vi "WHD_VEten_0.1.2_WS_BIDIREC_update_it-0065.vi"() -> ()   [LabVIEW 2015]
uses:
  <vilib>/LabVIEW Targets/FPGA/cRIO/shared/nicrio_ModuleControls/nicrio_cRIO-9234_DataRatesRing2.ctl
  <vilib>/RTwatchdog.llb/Watchdog expiration actions.ctl
  <vilib>/userdefined/High Color/nirio_resource_hc.ctl
  <vilib>/FPGAPlugInAG/cRIO-9031/niLvFpga_Open_cRIO-9031.vi
  <vilib>/Utility/file.llb/Write Delimited Spreadsheet (string).vi
  <vilib>/FPGAPlugInAG/cRIO-9031/niLvFpga_Run_cRIO-9031.vi
  <vilib>/Utility/error.llb/Error Cluster From Error Code.vi
  <vilib>/rvi/errors/niLvFpgaAdjustHostInterfaceError.vi
  <vilib>/rvi/interface/common/niFpgaWaitOnOcc.vi
  <vilib>/FPGAPlugInAG/cRIO-9031/niLvFpga_Reset_cRIO-9031.vi
  <vilib>/FPGAPlugInAG/cRIO-9031/niLvFpga_Close_cRIO-9031.vi
  <vilib>/rvi/interface/nirviOpenFPGA/nirviOpenFPGA.xnode
  FPGA Bitfiles/W&RDEuskotrenIBA_FPGATarget2_FPGA8a2wsBIdirec_MwruJOs6jio.lvbitx
  <vilib>/rvi/interface/nirviMethod/nirviMethod.xnode
  <vilib>/rvi/interface/nirviReadWriteControl/nirviReadWriteControl.xnode
  <vilib>/rvi/interface/nirviCloseFPGA/nirviCloseFPGA.xnode
  <vilib>/NI_Real-Time Target Support.lvlib
  AURA_Wheel/Json2Labv.lvlib
  AURA_Wheel/AuraWheelAPI/AuraWheel.lvlib
  NiFpgaLv.dll
  <vilib>/rvi/errors/niLvFpgaMergeErrorWithErrorCode.vi
  <vilib>/nisyscfg/nisyscfg.lvlib
  <vilib>/FPGAPlugInAG/cRIO-9031/niLvFpga_ConfigureFifo_cRIO-9031.vi
  <vilib>/FPGAPlugInAG/cRIO-9031/niLvFpga_StartFifo_cRIO-9031.vi
  <vilib>/FPGAPlugInAG/cRIO-9031/niLvFpga_ReadFifo_cRIO-9031.vi
  <vilib>/FPGAPlugInAG/cRIO-9031/niLvFpga_StopFifo_cRIO-9031.vi
panel:
  out "hora max subida datos":string
  out "hora subida datos":string
  in  "LIMITE MIN":dbl
  in  "LIMITE MAX":dbl
  in  "Parametros AuraWheel Health":string[](array[string])=["nem1234", "test_rest", "http://api.aurawheel.dev/services/devices/status"]
  out "Problema WS":bool
  out "Direccion 0?":bool
  out "Boton Adquirir?":bool
  out "RuedaDetectada2?":bool=TRUE
  out "RuedaDetectada1?":bool=TRUE
  in  "Timeout ruedas":dbl
  in  "Borrar archivos\nadquisicion con error":bool
  out "Watchdog config":T1={"reset"=FALSE, "occurrence"=FALSE, "trigger protocol"=enum."active high", "trigger line"=enum."none", "disable watchdog on VI exit"=TRUE}
  in  "Disable watchdog?":bool
  in  "Reset watchdog?":bool
  in  "Leer config RFID NEM":bool
  in  "bytes to read":i32
  in  "DeviceAddress":u8
  in  "timeout ms (60000)":i32
  in  "Max archivos":u32=2
  in  "Bytes libre despues de borrar":u32=2
  in  "Bytes min libre":u32=2
  in  "Nº de acelerómetros":i32
  in  "Nº inductivos":i32
  in  "Offset_rueda WS 1":fxp<+/-,24,-4>=0.004999998956918716 format="%.27g"
  out "TAGs_AURAwheel":string[][](array[string])
  out "Plataformas?":bool
  out "Nº Ejes":i32[](array[numeric])
  out "Nº UTs":i32
  out "it-read-LR6":i32[](array[numeric])
  out "it-LR6":i32
  out "RFID_LR6_Error":errorcluster
  out "Series_flota":string[](array[string])
  out "Tabla_flota":string[][](array[string])
  out "Puntos medios de las ventanas":dbl[][](array[numeric])
  out "configuration file path":path=path "c:/Parametros.cfg"
  in  "IP synchr":string
  out "data":cluster{"status":string}
  out "confRFID":path=path "c:/RFID/TAGS.csv"
  out "TAGS leidos":path=path "c:/RFID/TAGS.csv"
  in  "Use Aura?":bool
  in  "Parametros AuraWheel":string[](array[string])
  in  "Parámetros acelerómetros":dbl[](array[numeric])
  in  "Tiempo de adquisicion":dbl=10.0
  in  "Adquirir":bool
  out "Fin":bool
  out "Contador":i32=1
  out "Path TEST":path=path "c:/TEST"
  out "Fallo det presencia":bool
  out "Path_Borrar":path=path "c:/Trenes"
  out "Longitud de la unidad":dbl
  out "Bucle Espera":i32
  out "Aviso no detección":string
  out "Time to Acquire Block (ms)":i32
  out "Distancia de acelerómetros":dbl[](array[numeric])
  out "Block Size":u32
  out "Distancias generales":dbl[](array[numeric])
  in  "Reset del controlador":bool
  in  "Configuración":bool
  in  "Parar la aplicación":bool
  out "RFID":bool=TRUE
  out "date/time string":string
  out "Timeout ruedas":bool
  out "Tiempo":dbl
  out "Inicio pasada":timestamp
  out "Ultimo TEST":timestamp
  out "Fuente":bool=TRUE
  out "Estado":string
  out "RFID_ID":refnum<k5>
  out "DC OK":string
  out "Aviso temperatura":string
  in  "Tab Control":T2(tab)=enum."Parámetros"
  out "V (m/s)":dbl
  out "Temperatura (ºC)":dbl
  out "Max RMS Ruedas":dbl[][](array[numeric])
  out "result":bool
  out "TAGs":string[](array[string])
  out "Parar":bool
  out "TAGs LR6":string[](array[string])
  out "TAGs HEX":string[](array[string])
  out "Waveform Graph":sgl[][](graph)
  out "Nombre de archivo":path[](array[path])
  out "Tiempo de paso (s)":dbl
  out "Tiempo extra de adquisición (s)":dbl
  out "Número de ejes detectados":i32
  out "Buffer Underflow":bool
  out "Buffer Overflow":bool
  out "Disco Duro Disponible (bytes)":i64
  out "created path":path
  out "Nº Ruedas 1":i32
  out "NºRuedas 2":i32
  out "deleted portion":sgl[](array[numeric])
  out "deleted portion 2":sgl[](array[numeric])
  out "Ejes_convoy":i32
  out "T fuera rango":bool
  in  "Frecuencia de muestreo (Hz)":dbl=25600.0
  in  "Escaneos de la FIFO por canal":u32=5000
  in  "Tiempo extra al detector de paso (s)":dbl=1.0
  in  "dt RMS":dbl=256.0
  in  "Frecuencia de muestreo y módulo CRIO":T3=2 items=["51.200 kS/s (NI 9234)"=1, "25.600 kS/s (NI 9234)"=2, "17.067 kS/s (NI 9234)"=3, "12.800 kS/s (NI 9234)"=4, "10.240 kS/s (NI 9234)"=5, "8.533 kS/s (NI 9234)"=6, "7.314 kS/s (NI 9234)"=7, "6.400 kS/s (NI 9234)"=8, "5.689 kS/s (NI 9234)"=9, "5.120 kS/s (NI 9234)"=10, "4.654 kS/s (NI 9234)"=11, "4.267 kS/s (NI 9234)"=12, "3.938 kS/s (NI 9234)"=13, "3.657 kS/s (NI 9234)"=14, "3.413 kS/s (NI 9234)"=15, "3.200 kS/s (NI 9234)"=16, "3.012 kS/s (NI 9234)"=17, "2.845 kS/s (NI 9234)"=18, "2.695 kS/s (NI 9234)"=19, "2.560 kS/s (NI 9234)"=20, "2.438 kS/s (NI 9234)"=21, "2.328 kS/s (NI 9234)"=22, "2.226 kS/s (NI 9234)"=23, "2.133 kS/s (NI 9234)"=24, "2.048 kS/s (NI 9234)"=25, "1.969 kS/s (NI 9234)"=26, "1.896 kS/s (NI 9234)"=27, "1.829 kS/s (NI 9234)"=28, "1.765 kS/s (NI 9234)"=29, "1.707 kS/s (NI 9234)"=30, "1.652 kS/s (NI 9234)"=31]
  in  "Puerto RFID":u16=2189
  in  "IP RFID":string="192.168.106.99"
  in  "Offset_rueda WS 2":fxp<+/-,24,-4>=0.004999998956918716 format="%.27g"
  in  "Count(mSec)":u32=2
  in  "LR6 IP address":string="192.168.106.94"
  in  "Port LR6":u16=2001
  in  "RFID NEM on?":bool
  in  "RFID LR6 on?":bool
  in  "Canal cero WS1?":bool
  in  "Canal cero WS2":bool
  out "Parámetros":bool=TRUE
  out "Distacias y medidas de dispositivos":bool=TRUE
  out "RFID_Error":errorcluster
  out "error FPGA":errorcluster
  out "error manipulacion archivos":errorcluster
  out "Unidades y ejes":bool=TRUE
  out "RFID":bool=TRUE
  out "error AURA":errorcluster
  out "Response headers":string
  in  "Array":path[](array[path])=[path "c:/Trenes_prueba/0207_2013-09-24_19-09-42_0.bin", path "c:/Trenes_prueba/0096_2013-10-30_18-13-14_0.bin", path "c:/Trenes_prueba/0001_2013-06-05_13-06-23_0.bin"]
  out "Numeric 3":i32
  in  "Digital?":bool=TRUE
  # "Funciona?"
  # "Última detección de unidad"
  # "Error!!"
  # "Estado de la memoria"
  # "Parámetros de muestreo"
  # "Parámetros de adquisición"
  # "Parámetros de procesado"
  # "Cambio Fecha y Hora"
  # "Cargar datos de configuración"
  # "Errores!!"
  # "WRD_MEX\nWRD_ZAR"
  # "0 tagMexInit\n1 tagMexFin\n\n0 tag1\n1 tag2"
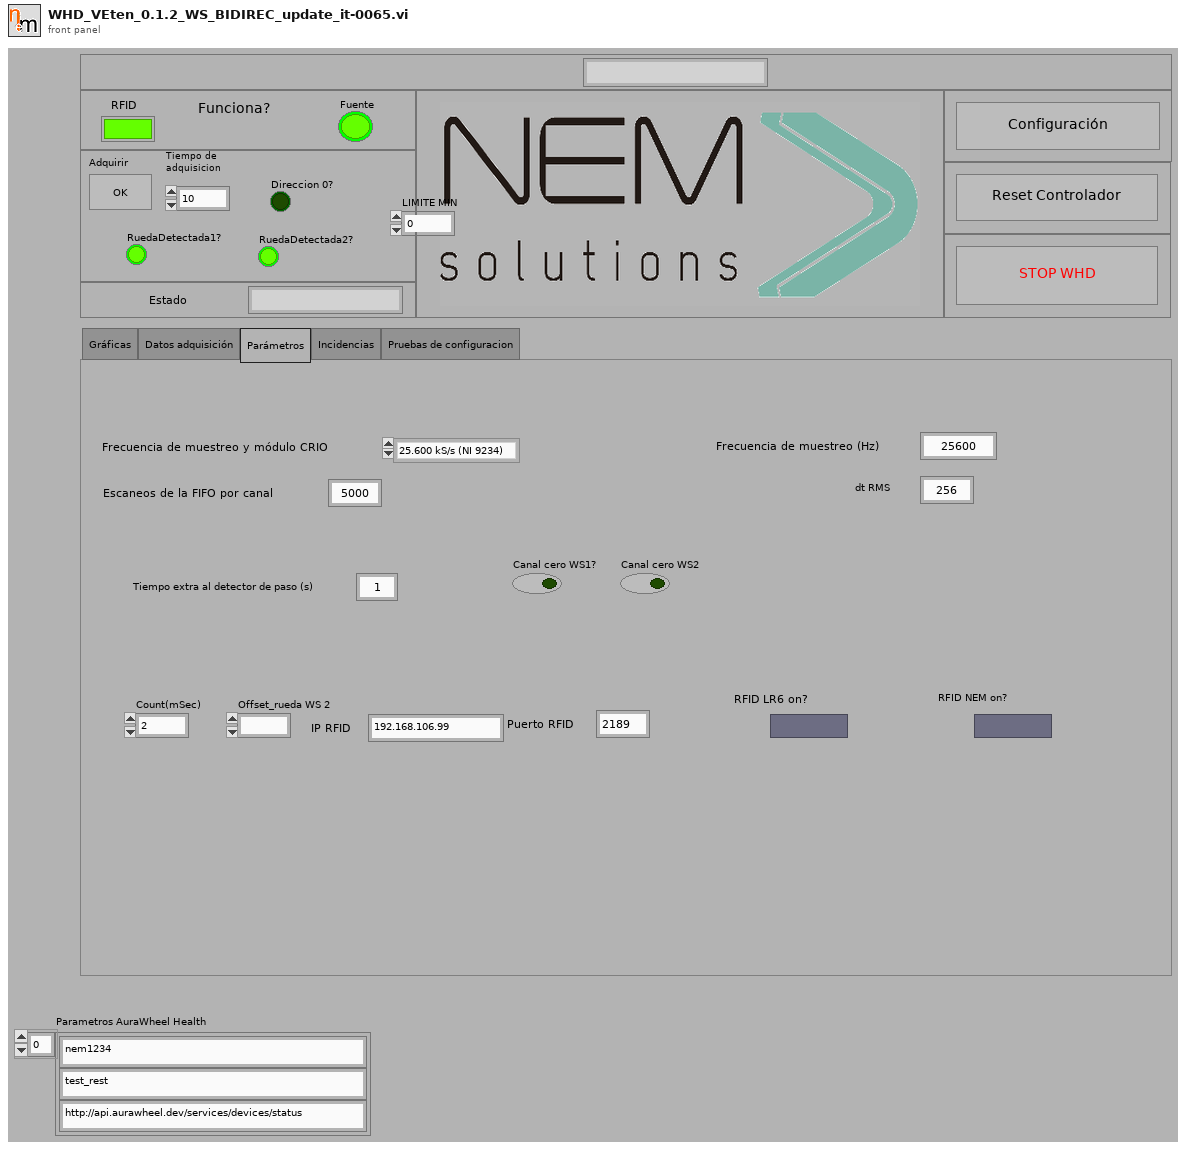
[diagram p1: front panel]
types:
  T1 = typedef "Watchdog expiration actions.ctl" = cluster{"reset":bool, "occurrence":bool, "trigger protocol":enum16{"active high", "active low", "open collector"}, "trigger line":enum16{"none", "line 0", "line 1", "line 2", "line 3", "line 4", "line 5", "line 6", "line 7", "SMB line 0"}, "disable watchdog on VI exit":bool}
  T2 = enum32{"Gráficas", "Datos adquisición", "Parámetros", "Incidencias", "Pruebas de configuracion"}
  T3 = typedef "nicrio_cRIO-9234_DataRatesRing2.ctl" = u8
  T4 = typedef "nirio_resource_hc.ctl" = tag
  T5 = enum16{"Standard", "Buffered", "CRLF", "Immediate"}
  T6 = enum16{"open", "replace", "create", "open or create", "replace or create", "replace or create with confirmation"}
  T7 = enum16{"big-endian, network order", "native, host order", "little-endian"}
  T8 = cluster{"error IO":errorcluster, bool[], u32[], string[], dbl[]}
  T9 = cluster{"g_ts":dbl, "p_sp":dbl, "p_tp":dbl, "p_tg":cluster{"tg_n":dbl, "tg_t":string}[], "p_ax":cluster{"ax_n":dbl, "ax_sp":dbl, "ax_wh":cluster{"wh_p":dbl, "wh_a1":dbl, "wh_a2":dbl, "wh_a3":dbl, "wh_a4":dbl}[]}[]}
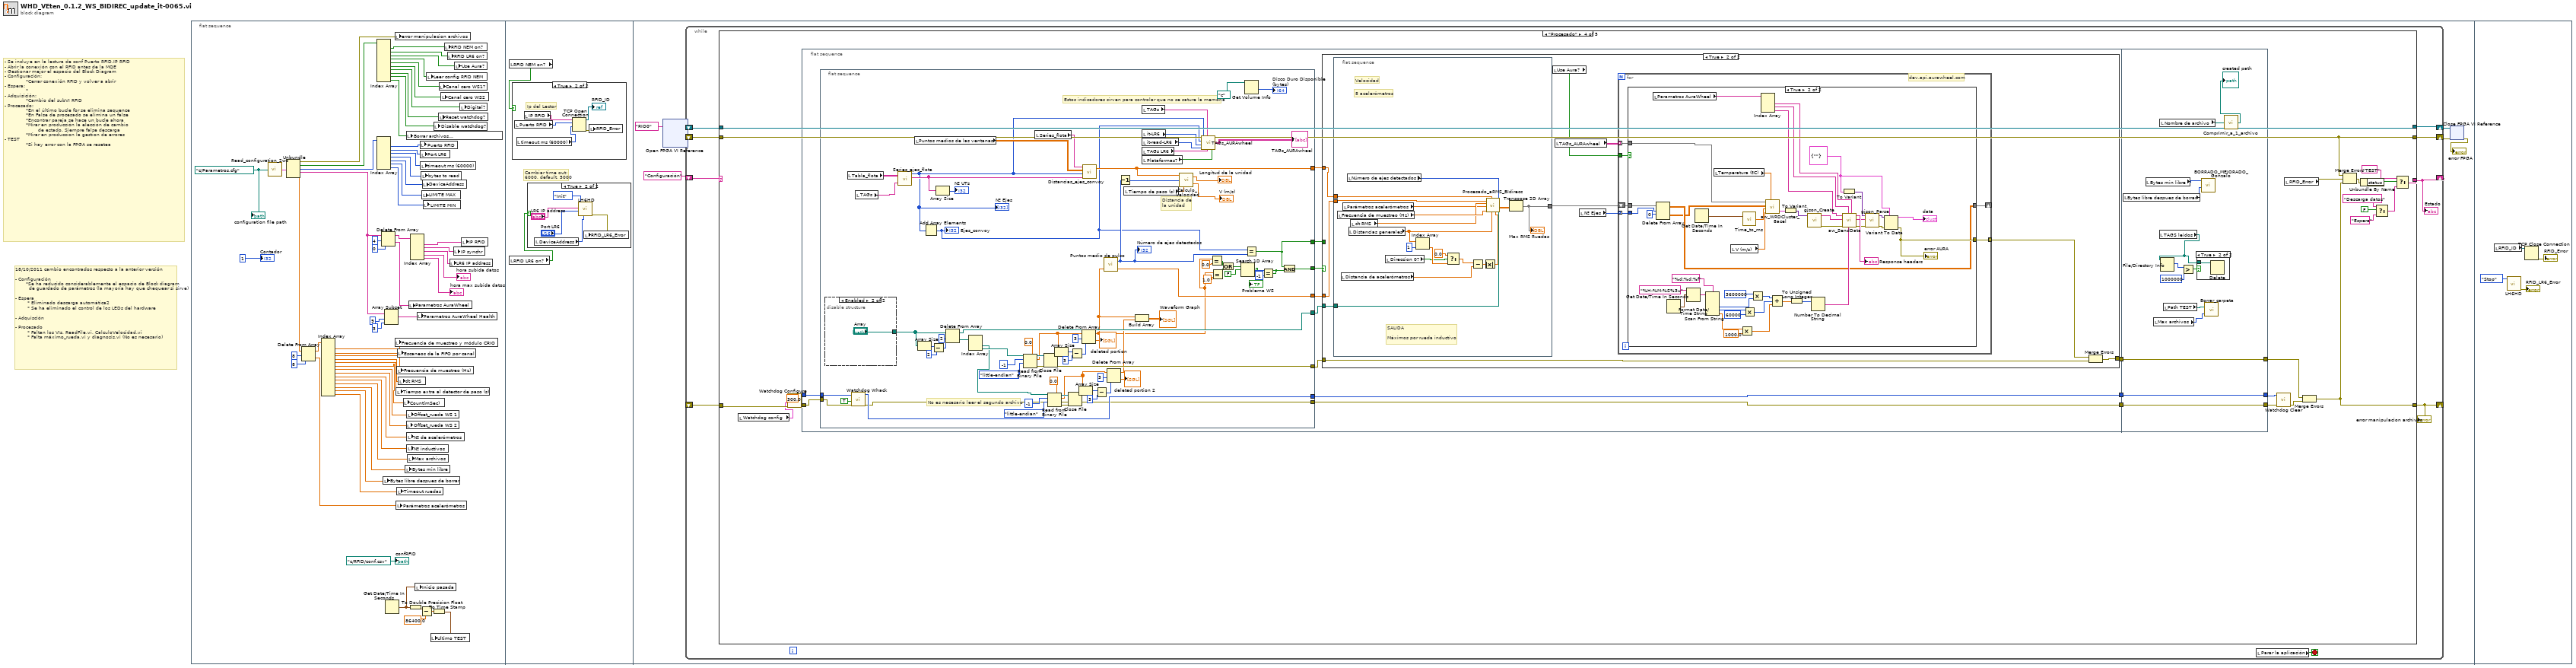
[diagram p0: block diagram]
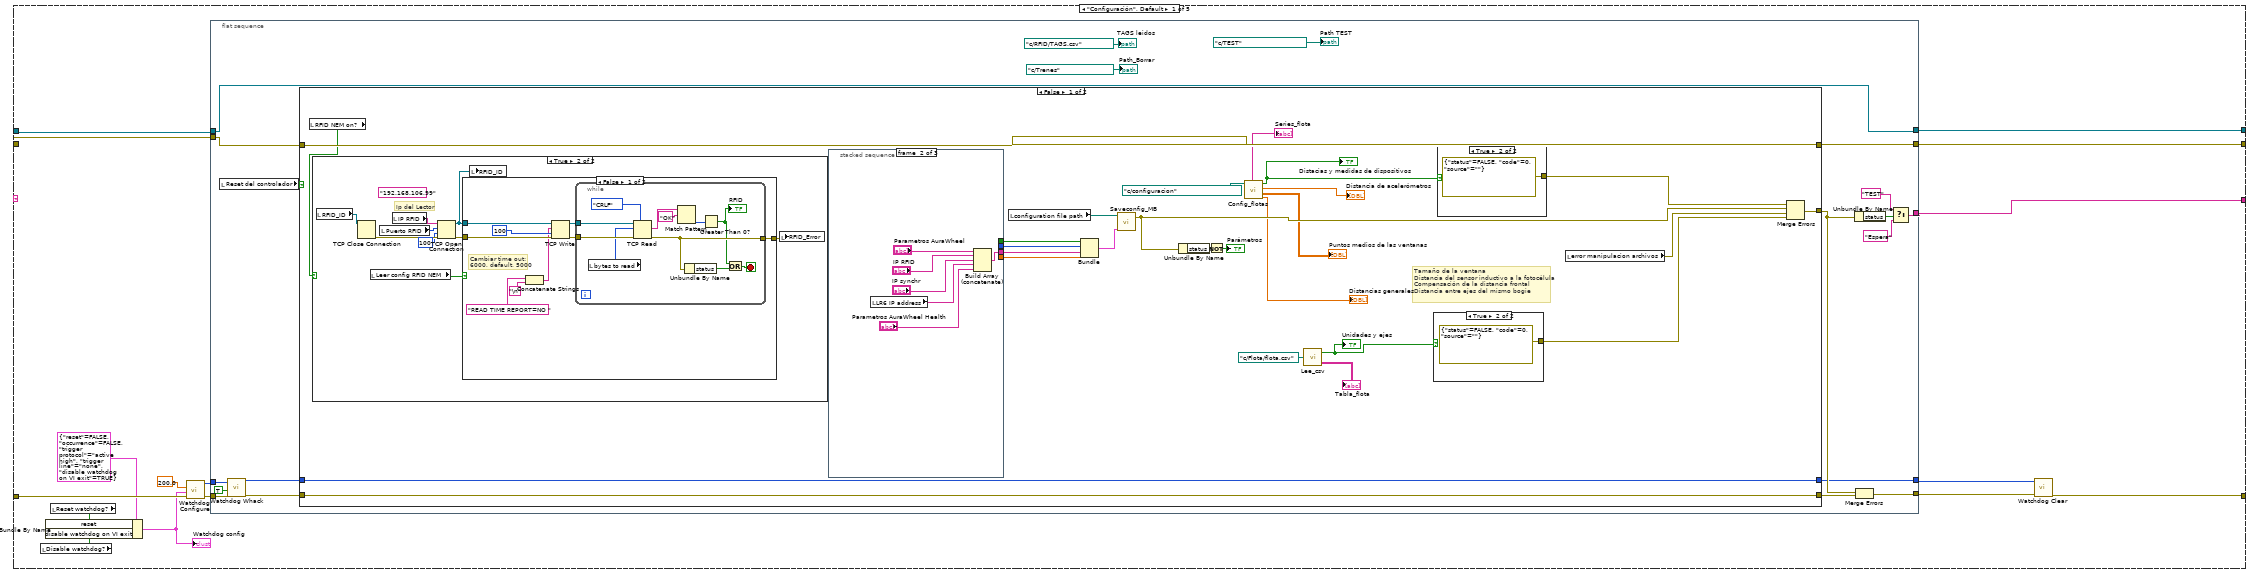
[diagram p4: hidden frame]
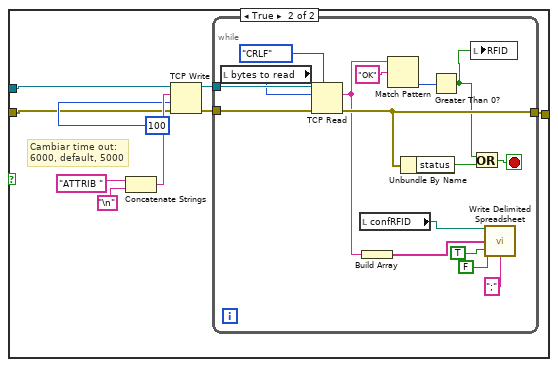
[diagram p6: hidden frame]
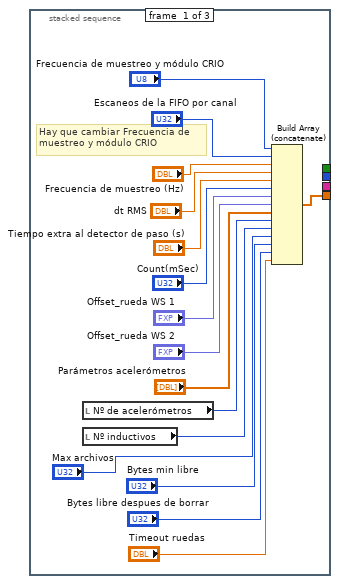
[diagram p7: hidden frame]
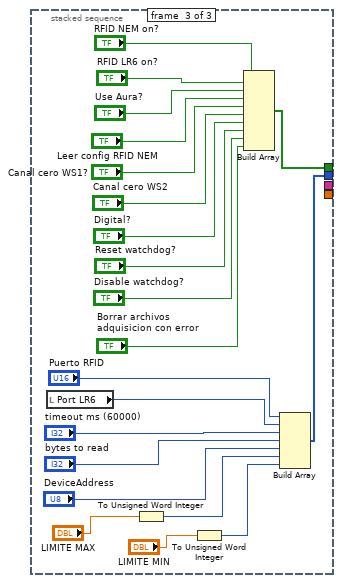
[diagram p8: hidden frame]
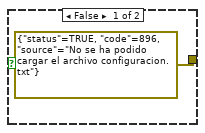
[diagram p9: hidden frame]
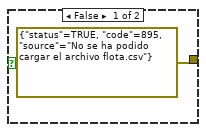
[diagram p10: hidden frame]
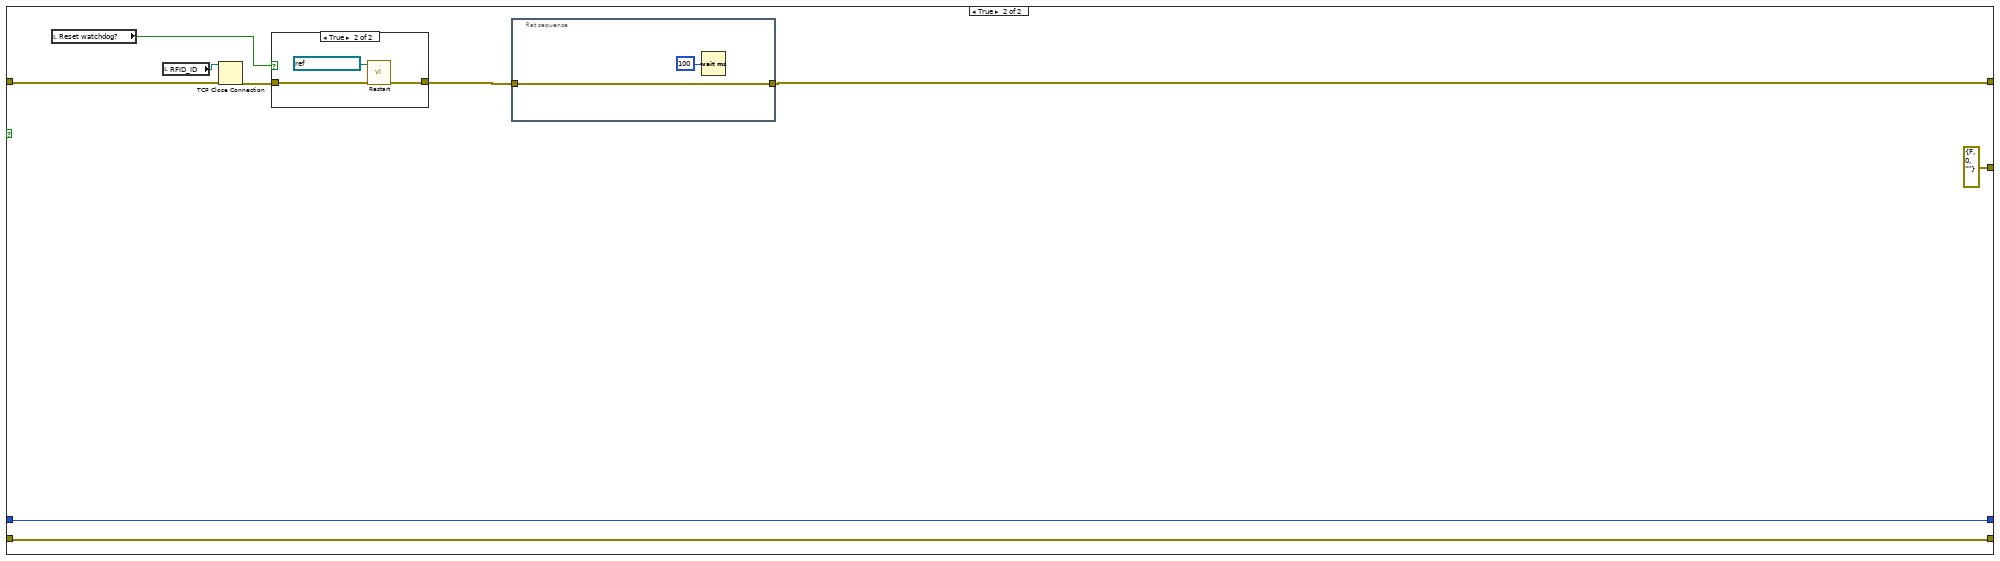
[diagram p11: hidden frame]
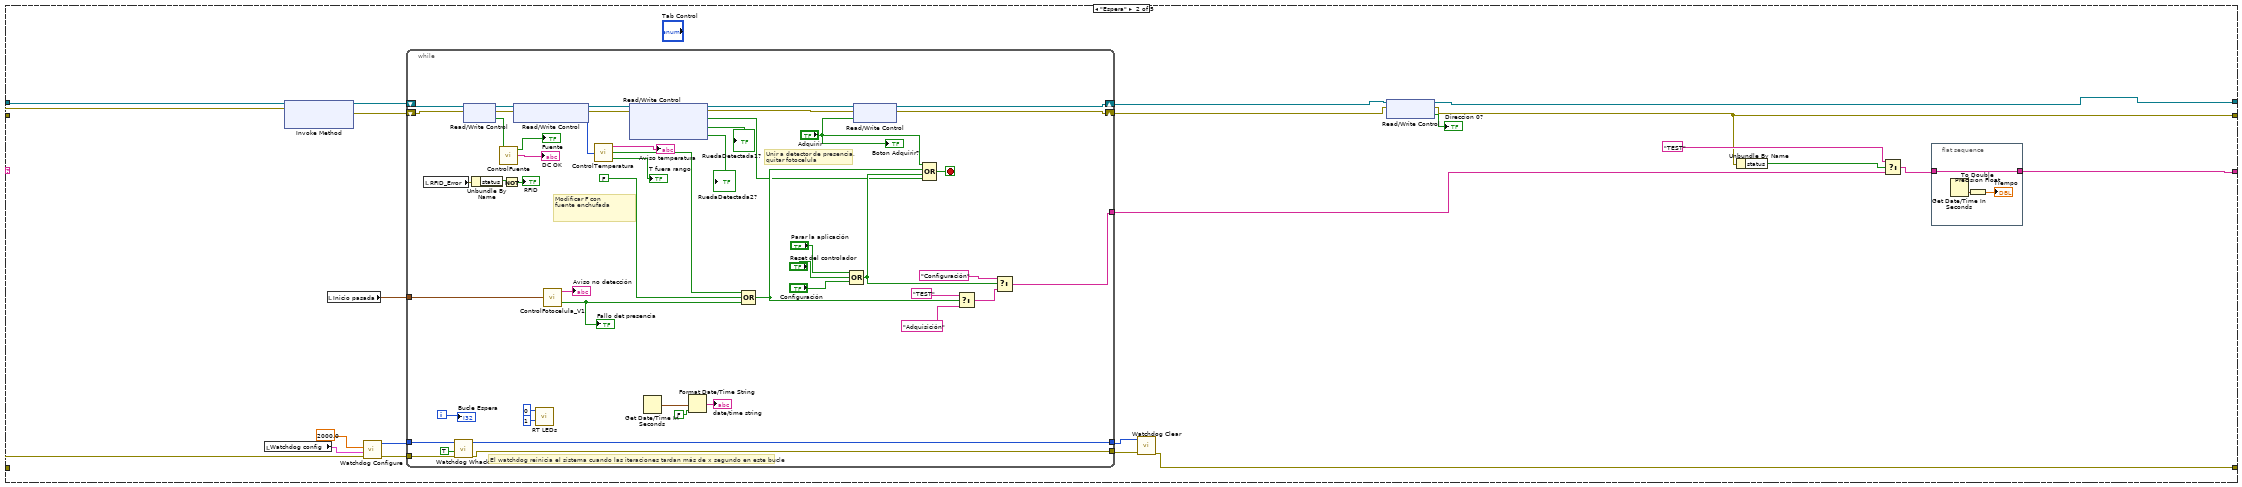
[diagram p13: hidden frame]
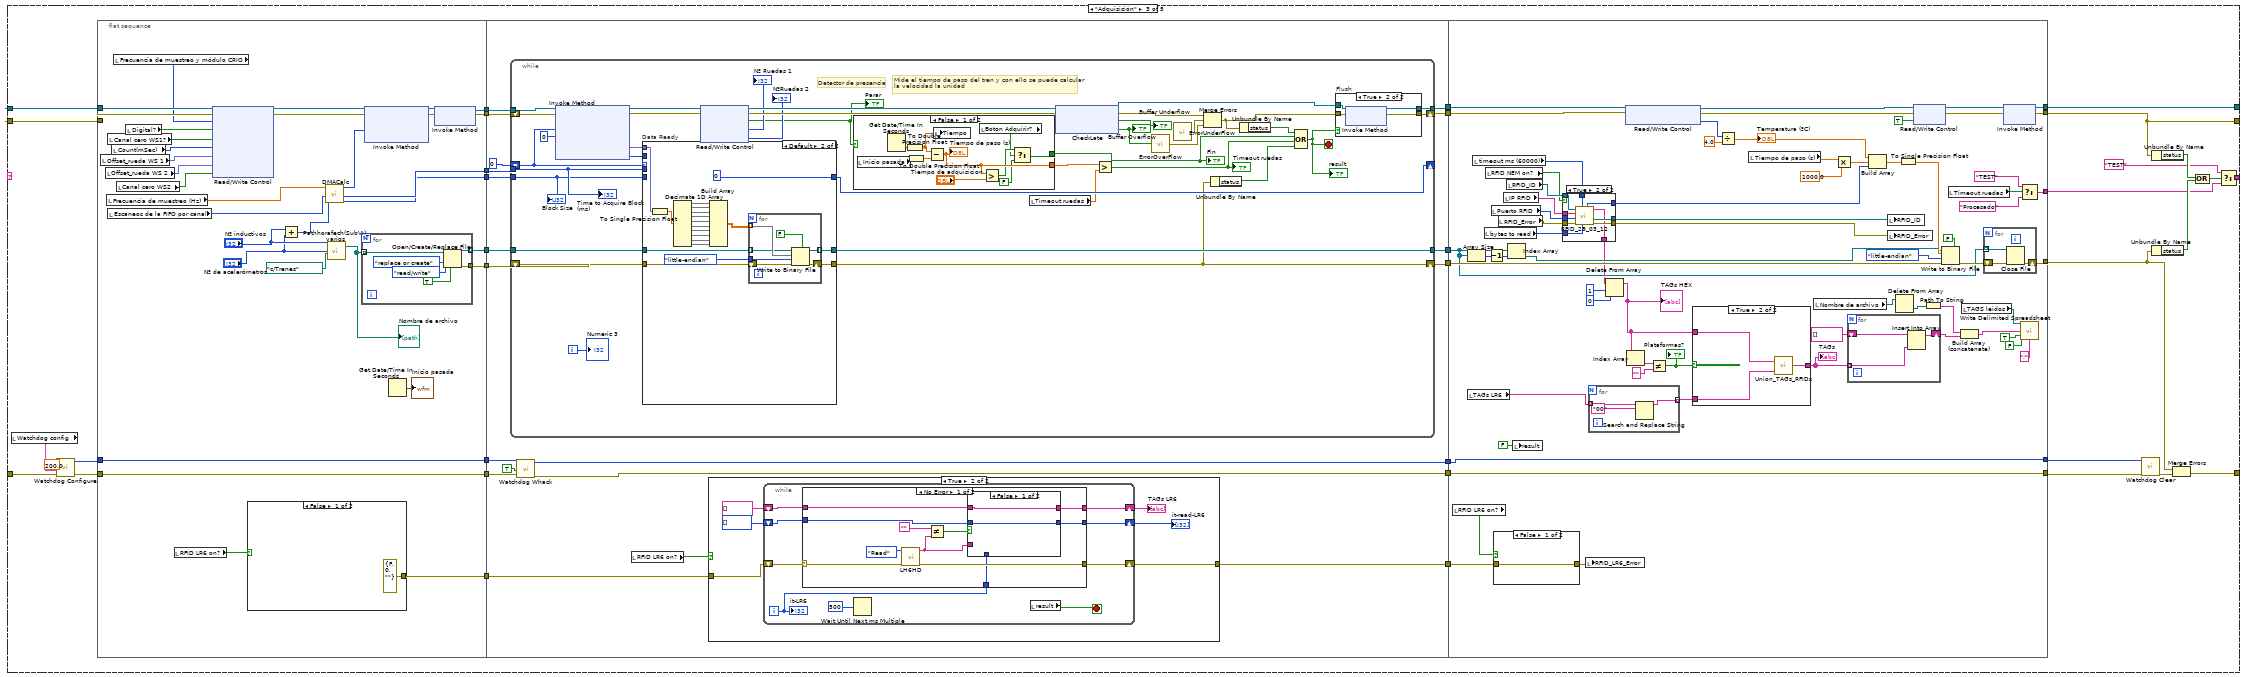
[diagram p14: hidden frame]
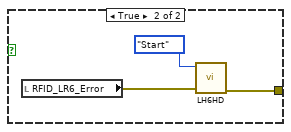
[diagram p15: hidden frame]
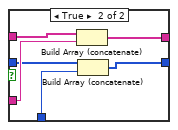
[diagram p17: hidden frame]
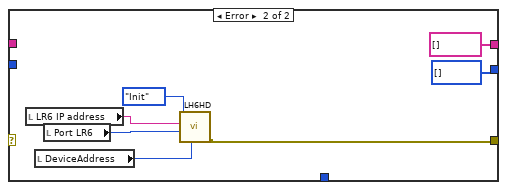
[diagram p18: hidden frame]
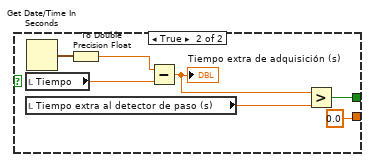
[diagram p19: hidden frame]
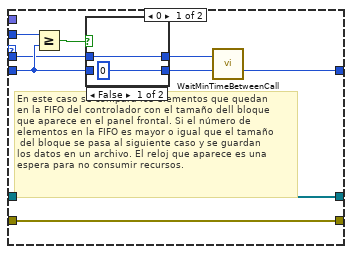
[diagram p20: hidden frame]
diagram:
  # "18/10/2011 cambio encontrados respecto a la anterior versión\n\n- Configuración\n       *Se ha reducido considerablemente el espacio de Block diagram\n         de guardado de parámetros (la mayoría hay que chequear si sirve)\n\n- Espera\n        * Eliminado descarga automática2\n        * Se ha eliminado el control de los LEDs del hardware\n       \n- Adquisción\n\n- Procesado\n        * Faltan los VIs, ReadFile.vi, CalculoVelocidad.vi\n        * Falta máximo_rueda.vi y diagnosis.vi (No es necesario)"
  # "- Se incluye en la lectura de conf Puerto RFID,IP RFID\n- Abrir la conexión con el RFID antes de la MQE\n- Gestionar mejor el espacio del Block Diagram\n- Configuración:\n              *Cerrar conexión RFID y volver a abrir\n- Espera:\n              *\n- Adquisición:\n              *Cambio del subVI RFID\n- Procesado:\n              *En el último bucle for se elimina sequence\n              *En False de procesado se elimina un false\n              *Encontrar pareja se hace un bucle ahora\n              *Mirar en producción la elección de cambio\n                      de estado. Siempre false descarga \n              *Mirar en produccion la gestion de errores\n- TEST\n              *Si hay error con la FPGA se resetea"
  n1 = flat-sequence {
    frame #0 {
      w45 = path "c:/Parametros.cfg" ("configuration file path")
      n2 = call "Read_configuration_2ws.vi"("configuration file path"=w45) -> ("output cluster"=w44:T8)
      n3 = Unbundle(w44) -> ("error IO"=w49:errorcluster, w48:bool[], w47:u32[], w8:string[], w42:dbl[])
      n4 = Delete From Array(array=w42, length=8, index=8) -> (deleted portion=w38:dbl[], array with subset deleted=w41:dbl[])
      n5 = Index Array(array=w41) -> (element #1=w56:dbl, element #2=w55:dbl, element #3=w54:dbl, element #4=w53:dbl, element #5=w52:dbl, element #6=w26:dbl, element #7=w25:dbl, element #8=w32:dbl, element #9=w24:dbl, element #10=w23:dbl, element #11=w22:dbl, element #12=w21:dbl, element #13=w20:dbl, element #14=w9:dbl)  [unwired: 14 in]
      n6 = Index Array(array=w48) -> (element #1=w51:bool, element #2=w50:bool, element #3=w37:bool, element #4=w16:bool, element #5=w15:bool, element #6=w14:bool, element #7=w13:bool, element #8=w12:bool, element #9=w11:bool, element #10=w10:bool)  [unwired: 10 in]
      n7 = Index Array(array=w47) -> (element #1=w43:u32, element #2=w27:u32, element #3=w19:u32, element #4=w18:u32, element #5=w17:u32, element #6=w4:u32, element #7=w3:u32)  [unwired: 7 in]
      n8 = Delete From Array(array=w8, length=4, index=0) -> (deleted portion=w30:string[], array with subset deleted=w36:string[])
      n9 = local write "Bytes libre despues de borrar"(w20) -> ()
      n10 = Array Subset(array=w8, index=9, length=3 ("index")) -> (w7:string[])
      n11 = Get Date/Time In Seconds() -> (seconds since 1Jan1904=w58:timestamp)
      n12 = local write "error manipulacion archivos"(w49) -> ()
      n13 = local write "Frecuencia de muestreo y módulo CRIO"(w56) -> ()
      n14 = local write "Parámetros acelerómetros"(w38) -> ()
      n15 = local write "Tiempo extra al detector de paso (s)"(w52) -> ()
      n16 = local write "Frecuencia de muestreo (Hz)"(w54) -> ()
      n17 = local write "Timeout ruedas"(w9) -> ()
      n18 = local write "Escaneos de la FIFO por canal"(w55) -> ()
      n19 = local write "dt RMS"(w53) -> ()
      n20 = local write "Count(mSec)"(w26) -> ()
      n21 = local write "Bytes min libre"(w21) -> ()
      n22 = local write "Borrar archivos\nadquisicion con error"(w10) -> ()
      n23 = local write "Offset_rueda WS 2"(w32) -> ()
      n24 = local write "Offset_rueda WS 1"(w25) -> ()
      n25 = local write "Nº de acelerómetros"(w24) -> ()
      n26 = local write "Nº inductivos"(w23) -> ()
      n27 = local write "Max archivos"(w22) -> ()
      n28 = local write "Parametros AuraWheel"(w30) -> ()
      n29 = To Double Precision Float(number=w58) -> (double precision float=w60:dbl)
      n30 = Index Array(array=w36) -> (element #1=w29:string, element #2=w31:string, element #3=w28:string, element #4=→"hora subida datos":string, element #5=→"hora max subida datos":string)  [unwired: 5 in]
      n31 = local write "Inicio pasada"(w58) -> ()
      n32 = local write "Parametros AuraWheel Health"(w7) -> ()
      n33 = local write "Puerto RFID"(w43) -> ()
      n34 = Subtract(x=w60, y=86400.0) -> (x-y=w59:dbl)
      n35 = local write "Port LR6"(w27) -> ()
      n36 = local write "timeout ms (60000)"(w19) -> ()
      n37 = local write "bytes to read"(w18) -> ()
      n38 = local write "LIMITE MAX"(w4) -> ()
      n39 = local write "DeviceAddress"(w17) -> ()
      n40 = local write "LIMITE MIN"(w3) -> ()
      n41 = local write "Leer config RFID NEM"(w16) -> ()
      n42 = To Time Stamp(1:w59) -> (0:w57:timestamp)
      n43 = local write "Ultimo TEST"(w57) -> ()
      n44 = local write "Disable watchdog?"(w11) -> ()
      n45 = local write "Reset watchdog?"(w12) -> ()
      n46 = local write "Canal cero WS1?"(w15) -> ()
      n47 = local write "Canal cero WS2"(w14) -> ()
      n48 = local write "RFID NEM on?"(w51) -> ()
      n49 = local write "RFID LR6 on?"(w50) -> ()
      n50 = local write "LR6 IP address"(w28) -> ()
      n51 = local write "IP synchr"(w31) -> ()
      n52 = local write "Use Aura?"(w37) -> ()
      n53 = local write "Digital?"(w13) -> ()
      n54 = local write "IP RFID"(w29) -> ()
      "Contador" <- 1
      "confRFID" <- path "c:/RFID/conf.csv" ("file path (use dialog)")
      "configuration file path" <- w45
    }
    frame #1 {
      # "Cambiar time out:\n6000, default, 5000"
      n55 = local read "RFID NEM on?"() -> (w63:bool)
      n56 = local read "RFID LR6 on?"() -> (w62:bool)
      n57 = case shown="True" w63 {
        frame False {
        }
        frame True {
          # "Ip del Lector"
          n58 = local read "Puerto RFID"() -> (w71:u16)
          n59 = local read "timeout ms (60000)"() -> (w69:i32)
          n60 = local read "IP RFID"() -> (w72:string)
          n61 = TCP Open Connection(address=w72, remote port or service name=w71, timeout ms (60000)=w69) -> (connection ID=→"RFID_ID":refnum<k5>, error out=w70:errorcluster)  [unwired: 1 in, 1 out]
          n62 = local write "RFID_Error"(w70) -> ()
        }
      }
      n63 = case shown="True" w62 {
        frame False {
        }
        frame True {
          n64 = local read "DeviceAddress"() -> (w64:u8)
          n65 = call "LH6HD.vi"("DeviceAddress"=w64, "Reader Port"="Port LR6", "IP Address"="LR6 IP address", "Action"=enum16{"Init", "Start", "Read", "Stop", "Exit"}."Init") -> ("error out"=w68:errorcluster)  [unwired: 6 in, 1 out]
          n66 = local write "RFID_LR6_Error"(w68) -> ()
        }
      }
    }
    frame #2 {
      n67 = xnode "Open FPGA VI Reference"("resource name"=T4 "RIO0") -> ("FPGA VI Reference Out"=w80:refnum<k20>, "error out"=w79:errorcluster)  [unwired: 1 in]
      n68 = while {
        shift-right: [w84] -> _
        shift-left: "Configuración" -> [w89]
        shift-right: [w82] -> w76
        shift-left: w80 -> [w88]
        shift-right: [w81] -> w75
        shift-left: w79 -> [w87]
        shift-right: [w86] -> _
        shift-left: _ -> [w85]
        stop <- w83 stop-if-true
        n69 = case shown="\"Procesado\"" w89 {
          tunnel: [w104 w281 w357 w691 w921] -> w84
          tunnel: [w103 w269 w371 w699 w920] -> w82
          tunnel: [w105 w268 w372 w686 w918] -> w81
          tunnel: w88 -> [w102 w286 w379 w699 w920]
          tunnel: w87 -> [w101 w284 w378 w686 w919]
          tunnel: [w94 w275 w369 w689 w908] -> w86
          tunnel: w85 -> [w100 w280 w353 w685 w913]
          frame "Configuración", Default {
            n70 = local read "Disable watchdog?"() -> (w92:bool)
            n71 = local read "Reset watchdog?"() -> (w91:bool)
            n72 = Bundle By Name(cluster=T1 {"reset"=FALSE, "occurrence"=FALSE, "trigger protocol"=enum."active high", "trigger line"=enum."none", "disable watchdog on VI exit"=TRUE} ("expiration actions"), "reset"=w91, "disable watchdog on VI exit"=w92) -> (w90:T1)
            "Watchdog config" <- w90
            n73 = call <vilib>:"Watchdog Configure.vi"("error in (no error)"=w100, "expiration actions"=w90, "timeout (1 sec)"=200.0) -> ("error out"=w97:errorcluster, "watchdogID"=w98:u64)  [unwired: 3 in, 2 out]
            n74 = flat-sequence {
              tunnel: [w116] -> w105
              tunnel: [w124] -> w104
              tunnel: w102 -> [w117]
              tunnel: [w117] -> w103
              tunnel: [w119] -> w95
              tunnel: w101 -> [w114]
              tunnel: w98 -> [w112]
              tunnel: w97 -> [w111]
              tunnel: [w109] -> w96
              frame #0 {
                n75 = local read "Reset del controlador"() -> (w113:bool)
                n76 = call <vilib>:"Watchdog Whack.vi"("error in (no error)"=w111, "reset watchdog after expire? (F)"=TRUE, "watchdogID in"=w112) -> ("error out"=w107:errorcluster, "watchdogID out"=w108:u64)  [unwired: 2 in, 1 out]
                n77 = case shown="False" w113 {
                  tunnel: w114 -> [w151 w259]
                  tunnel: [w151 w258] -> w116
                  tunnel: [w137 errorcluster {"status"=FALSE, "code"=0, "source"=""} ("error IO")] -> w115
                  tunnel: [w129 w257] -> w109
                  tunnel: w108 -> [w129 w257]
                  tunnel: w107 -> [w128 w256]
                  tunnel: [w128 w256] -> w106
                  frame False {
                    # "Tamaño de la ventana\nDistancia del sensor inductivo a la fotocélula\nCompensación de la distancia frontal\nDistancia entre ejes del mismo bogie"
                    n78 = local read "RFID NEM on?"() -> (w127:bool)
                    n79 = case shown="True" w127 {
                      frame False {
                      }
                      frame True {
                        (unwired) "192.168.106.99" ("address")
                        # "Ip del Lector"
                        n80 = local read "RFID_ID"() -> (w159:refnum<k5>)
                        n81 = TCP Close Connection(connection ID=w159) -> (error out=w160:errorcluster)  [unwired: 2 in, 1 out]
                        n82 = local read "Leer config RFID NEM"() -> (w152:bool)
                        n83 = local read "Puerto RFID"() -> (w157:u16)
                        n84 = local read "IP RFID"() -> (w156:string)
                        n85 = TCP Open Connection(address=w156, remote port or service name=w157, timeout ms (60000)=100, error in (no error)=w160) -> (connection ID=w158:refnum<k5>, error out=w153:errorcluster)  [unwired: 1 out]
                        n86 = case shown="False" w152 {
                          tunnel: w158 -> [w169 w183]
                          tunnel: [w167 w181] -> w154
                          tunnel: w153 -> [w164 w182]
                          frame False {
                            # "Cambiar time out:\n6000, default, 5000"
                            n87 = Concatenate Strings("READ TIME REPORT=NO " ("data in"), "\n") -> (w161:string)
                            n88 = TCP Write(connection ID=w169, data in=w161, error in (no error)=w164, 9:100 ("timeout ms (25000)")) -> (connection ID out=w165:refnum<k5>, error out=w166:errorcluster)  [unwired: 1 out]
                            n89 = while {
                              tunnel: w166 -> [w179]
                              tunnel: w165 -> [w178]
                              tunnel: [w177] -> w167
                              stop <- w174 stop-if-true
                              n90 = local read "bytes to read"() -> (w170:i32)
                              n91 = TCP Read(connection ID=w178, bytes to read=w170, error in (no error)=w179, 7:T5."CRLF" ("mode (standard)")) -> (data out=w172:string, error out=w177:errorcluster)  [unwired: 1 in, 1 out]
                              n92 = Match Pattern(string=w172, regular expression="OK") -> (offset past match=w175:i32)  [unwired: 4 out]
                              n93 = Unbundle By Name(w177) -> ("status"=w173:bool)
                              n94 = Greater Than 0?(x=w175) -> (x > 0?=w171:bool)
                              "RFID" <- w171
                              n95 = Or(x=w171, y=w173) -> (x .or. y?=w174:bool)
                            }
                          }
                          frame True {
                            # "Cambiar time out:\n6000, default, 5000"
                            n96 = Concatenate Strings("ATTRIB " ("data in"), "\n") -> (w189:string)
                            n97 = TCP Write(connection ID=w183, data in=w189, error in (no error)=w182, 9:100 ("timeout ms (25000)")) -> (connection ID out=w186:refnum<k5>, error out=w185:errorcluster)  [unwired: 1 out]
                            n98 = while {
                              tunnel: w185 -> [w204]
                              tunnel: w186 -> [w203]
                              tunnel: [w202] -> w181
                              stop <- w199 stop-if-true
                              n99 = local read "bytes to read"() -> (w190:i32)
                              n100 = TCP Read(connection ID=w203, bytes to read=w190, error in (no error)=w204, 7:T5."CRLF" ("mode (standard)")) -> (data out=w193:string, error out=w202:errorcluster)  [unwired: 1 in, 1 out]
                              n101 = local read "confRFID"() -> (w192:path)
                              n102 = Build Array(w193) -> (w191:string[])
                              n103 = Match Pattern(string=w193, regular expression="OK") -> (offset past match=w200:i32)  [unwired: 4 out]
                              n104 = Unbundle By Name(w202) -> ("status"=w198:bool)
                              n105 = Greater Than 0?(x=w200) -> (x > 0?=w197:bool)
                              n106 = local write "RFID"(w197) -> ()
                              n107 = Or(x=w197, y=w198) -> (x .or. y?=w199:bool)
                              n108 = call-poly <vilib>:"Write Delimited Spreadsheet.vi"("file path (dialog if empty)"=w192, "1D data"=w191, "append to file? (F)"=FALSE ("transpose? (no:F)"), "transpose? (F)"=TRUE ("append to file? (new file:F)"), "delimiter (\\t)"=";" ("delimiter (\\t)")) -> ()  [unwired: 9 in, 2 out]
                            }
                          }
                        }
                        n109 = local write "RFID_ID"(w158) -> ()
                        n110 = local write "RFID_Error"(w154) -> ()
                      }
                    }
                    n111 = stacked-sequence {
                      tunnel: [w217 _ _] -> w141
                      tunnel: [_ w227 _] -> w140
                      tunnel: [_ _ w245] -> w142
                      tunnel: [_ _ w244] -> w143
                      frame #0 {
                        # "Hay que cambiar Frecuencia de\nmuestreo y módulo CRIO"
                        n112 = local read "Nº de acelerómetros"() -> (w211:i32)
                        n113 = local read "Nº inductivos"() -> (w210:i32)
                        n114 = Build Array (concatenate)("Frecuencia de muestreo y módulo CRIO", "Escaneos de la FIFO por canal", "Frecuencia de muestreo (Hz)", "dt RMS", "Tiempo extra al detector de paso (s)", "Count(mSec)", "Offset_rueda WS 1", "Offset_rueda WS 2", "Parámetros acelerómetros", w211, w210, "Max archivos", "Bytes min libre", "Bytes libre despues de borrar", "Timeout ruedas") -> (w217:dbl[])
                      }
                      frame #1 {
                        n115 = local read "LR6 IP address"() -> (w223:string)
                        n116 = Build Array (concatenate)("Parametros AuraWheel", "IP RFID", "IP synchr", w223, "Parametros AuraWheel Health") -> (w227:string[])
                      }
                      frame #2 {
                        n117 = local read "Port LR6"() -> (w241:u16)
                        n118 = To Unsigned Word Integer(number="LIMITE MAX") -> (unsigned 16bit integer=w230:u16)
                        n119 = To Unsigned Word Integer(number="LIMITE MIN") -> (unsigned 16bit integer=w228:u16)
                        n120 = Build Array("RFID NEM on?", "RFID LR6 on?", "Use Aura?", "Leer config RFID NEM", "Canal cero WS1?", "Canal cero WS2", "Digital?", "Reset watchdog?", "Disable watchdog?", "Borrar archivos\nadquisicion con error") -> (w244:bool[])
                        n121 = Build Array("Puerto RFID", w241, "timeout ms (60000)", "bytes to read", "DeviceAddress", w230, w228) -> (w245:i32[])
                      }
                    }
                    n122 = local read "configuration file path"() -> (w138:path)
                    n123 = Bundle(w143, w142, w140, w141) -> (w139:cluster{bool[], i32[], string[], dbl[]})  [unwired: 1 in]
                    n124 = call "Saveconfig_MB.vi"("configuration file path"=w138, "Configuracion"=w139) -> ("error out"=w146:errorcluster)  [unwired: 4 in]
                    n125 = Unbundle By Name(w146) -> ("status"=w147:bool)
                    n126 = Not(x=w147) -> (.not. x?=→"Parámetros":bool)
                    n127 = call "Config_flotas.vi"("file path (dialog if empty)"=path "c:/configuracion") -> ("Distancias generales"=→"Distancias generales":dbl[], "Puntos medios de las ventanas"=→"Puntos medios de las ventanas":dbl[][], "Distancia de acelerómetros"=→"Distancia de acelerómetros":dbl[], "Distacias y medidas de dispositivos"=w136:bool, "Series_flota"=→"Series_flota":string[])  [unwired: 3 in]
                    "Distacias y medidas de dispositivos" <- w136
                    n128 = call "Lee_csv.vi"("Path"=path "c:/Flota/flota.csv") -> ("Tabla_flota"=→"Tabla_flota":string[][], "Lectura_OK?"=w133:bool)
                    "Unidades y ejes" <- w133
                    n129 = case shown="True" w133 {
                      tunnel: [errorcluster {"status"=TRUE, "code"=895, "source"="No se ha podido cargar el archivo flota.csv"} ("error out") errorcluster {"status"=FALSE, "code"=0, "source"=""} ("error out")] -> w144
                      frame False {
                      }
                      frame True {
                      }
                    }
                    n130 = case shown="True" w136 {
                      tunnel: [errorcluster {"status"=TRUE, "code"=896, "source"="No se ha podido cargar el archivo configuracion.txt"} ("error out") errorcluster {"status"=FALSE, "code"=0, "source"=""} ("error out")] -> w149
                      frame False {
                      }
                      frame True {
                      }
                    }
                    n131 = local read "error manipulacion archivos"() -> (w145:errorcluster)
                    n132 = Merge Errors(w149, w146, w145, w144) -> (w137:errorcluster)
                  }
                  frame True {
                    n133 = local read "Reset watchdog?"() -> (w253:bool)
                    n134 = local read "RFID_ID"() -> (w261:refnum<k5>)
                    n135 = TCP Close Connection(connection ID=w261, error in (no error)=w259) -> (error out=w255:errorcluster)  [unwired: 2 out]
                    n136 = case shown="True" w253 {
                      tunnel: w255 -> [w262 w265]
                      tunnel: [w262 w264] -> w254
                      frame False {
                      }
                      frame True {
                        n137 = call <vilib>:"Restart.vi"("error in (no error)"=w265, "Session in"=refnum<k21> "localhost") -> ("error out"=w264:errorcluster)  [unwired: 7 in, 2 out]
                      }
                    }
                    n138 = flat-sequence {
                      tunnel: [w267] -> w258
                      tunnel: w254 -> [w267]
                      frame #0 {
                        n139 = Wait (ms)(milliseconds to wait=u32 100) -> ()  [unwired: 1 out]
                      }
                    }
                  }
                }
                n140 = Unbundle By Name(w115) -> ("status"=w125:bool)
                n141 = Merge Errors(w115, w106) -> (w119:errorcluster)
                n142 = Select(t="TEST", s=w125, f="Espera") -> (s? t:f=w124:string)
                "Path_Borrar" <- path "c:/Trenes" ("file path (use dialog)")
                "Path TEST" <- path "c:/TEST" ("file path (use dialog)")
                "TAGS leidos" <- path "c:/RFID/TAGS.csv" ("file path (use dialog)")
              }
            }
            n143 = call <vilib>:"Watchdog Clear.vi"("error in (no error)"=w95, "watchdogID in"=w96) -> ("error out"=w94:errorcluster)  [unwired: 5 in]
          }
          frame "Espera" {
            n144 = local read "Watchdog config"() -> (w274:T1)
            n145 = xnode "Invoke Method"("FPGA VI Reference In"=w286, "error in"=w284) -> ("FPGA VI Reference Out"=w285:refnum<k20>, "error out"=w283:errorcluster)  [unwired: 1 in]
            n146 = local read "Inicio pasada"() -> (w290:timestamp)
            n147 = call <vilib>:"Watchdog Configure.vi"("error in (no error)"=w280, "expiration actions"=w274, "timeout (1 sec)"=2000.0) -> ("error out"=w279:errorcluster, "watchdogID"=w278:u64)  [unwired: 3 in, 2 out]
            n148 = while {
              tunnel: [w312] -> w289
              shift-right: [w300] -> w270
              shift-left: w285 -> [w314]
              shift-right: [w299] -> w271
              shift-left: w283 -> [w313]
              tunnel: w290 -> [w317]
              tunnel: w279 -> [w297]
              tunnel: w278 -> [w298]
              tunnel: [w296] -> w277
              tunnel: [w295] -> w276
              i -> [w336]
              stop <- w343 stop-if-true
              # "Modificar F con\nfuente enchufada"
              # "Unir a detector de presencia,\nquitar fotocelula"
              # "El watchdog reinicia el sistema cuando las iteraciones tardan más de x segundo en este bucle"
              n149 = local read "RFID_Error"() -> (w320:errorcluster)
              n150 = call <vilib>:"Watchdog Whack.vi"("error in (no error)"=w297, "reset watchdog after expire? (F)"=TRUE, "watchdogID in"=w298) -> ("error out"=w295:errorcluster, "watchdogID out"=w296:u64)  [unwired: 2 in, 1 out]
              n151 = xnode "Read/Write Control"("FPGA VI Reference In"=w314, "error in"=w313) -> ("FPGA VI Reference Out"=w331:refnum<k20>, "error out"=w330:errorcluster, "DC OK"=w335:bool)
              n152 = Unbundle By Name(w320) -> ("status"=w318:bool)
              n153 = call "ControlFuente.vi"("DC OK 3"=w335) -> ("DC OK 2"=→"Fuente":bool, "DC OK"=→"DC OK":string)  [unwired: 1 out]
              n154 = Not(x=w318) -> (.not. x?=→"RFID":bool)
              n155 = xnode "Read/Write Control"("FPGA VI Reference In"=w331, "error in"=w330) -> ("FPGA VI Reference Out"=w326:refnum<k20>, "error out"=w325:errorcluster, "Chassis Temperature"=w333:i16)
              n156 = call <vilib>:"RT LEDs.vi"("State"=1, "LED Num"=0) -> ()  [unwired: 1 in, 5 out]
              n157 = call "ControlFotocelula_V1.vi"("Tiempo de entrada a espera"=w317) -> ("Aviso no detección"=→"Aviso no detección":string, "Boolean"=w323:bool)
              "Fallo det presencia" <- w323
              n158 = call "ControlTemperatura.vi"("Chassis Temperature"=w333) -> ("Aviso temperatura"=→"Aviso temperatura":string, "Boolean"=w327:bool, "T fuera rango"=→"T fuera rango":bool)
              n159 = xnode "Read/Write Control"("FPGA VI Reference In"=w326, "error in"=w325) -> ("FPGA VI Reference Out"=w316:refnum<k20>, "error out"=w315:errorcluster, "Detector de presencia"=w307:bool, "RuedaDetectada1?"=→"RuedaDetectada1?":bool, "RuedaDetectada2?"=→"RuedaDetectada2?":bool)
              n160 = Get Date/Time In Seconds() -> (seconds since 1Jan1904=w309:timestamp)
              n161 = Format Date/Time String(seconds (now)=w309, UTC format=FALSE) -> (date/time string=→"date/time string":string)  [unwired: 1 in]
              n162 = Compound Arithmetic op=OR(w327, FALSE ("value"), w323) -> (w324:bool)
              n163 = Compound Arithmetic op=OR("Parar la aplicación", "Reset del controlador", "Configuración") -> (w321:bool)
              n164 = xnode "Read/Write Control"("FPGA VI Reference In"=w316, "error in"=w315, "Fotocélula"="Adquirir") -> ("FPGA VI Reference Out"=w300:refnum<k20>, "error out"=w299:errorcluster)
              n165 = Compound Arithmetic op=OR("Adquirir", w324, w321, w307) -> (w343:bool)
              n166 = Select(t="TEST", s=w324, f="Adquisición") -> (s? t:f=w339:string)
              n167 = Select(t="Configuración", s=w321, f=w339) -> (s? t:f=w312:string)
              "Bucle Espera" <- w336
              "Boton Adquirir?" <- "Adquirir"
            }
            n168 = call <vilib>:"Watchdog Clear.vi"("error in (no error)"=w276, "watchdogID in"=w277) -> ("error out"=w275:errorcluster)  [unwired: 5 in]
            n169 = xnode "Read/Write Control"("FPGA VI Reference In"=w270, "error in"=w271) -> ("FPGA VI Reference Out"=w269:refnum<k20>, "error out"=w268:errorcluster, "Direccion 0?"=→"Direccion 0?":bool)
            n170 = Unbundle By Name(w268) -> ("status"=w288:bool)
            n171 = Select(t="TEST", s=w288, f=w289) -> (s? t:f=w282:string)
            n172 = flat-sequence {
              tunnel: [w292] -> w281
              tunnel: w282 -> [w292]
              frame #0 {
                n173 = Get Date/Time In Seconds() -> (seconds since 1Jan1904=w293:timestamp)
                n174 = To Double Precision Float(number=w293) -> (double precision float=→"Tiempo":dbl)
              }
            }
          }
          frame "Adquisición" {
            n175 = local read "Watchdog config"() -> (w354:T1)
            n176 = call <vilib>:"Watchdog Configure.vi"("error in (no error)"=w353, "expiration actions"=w354, "timeout (1 sec)"=200.0) -> ("error out"=w351:errorcluster, "watchdogID"=w352:u64)  [unwired: 3 in, 2 out]
            n177 = flat-sequence {
              tunnel: w378 -> [w407]
              tunnel: w379 -> [w408]
              tunnel: [w406] -> w368
              tunnel: [w405] -> w367
              tunnel: [w404] -> w366
              tunnel: [w403] -> w365
              tunnel: [w402] -> w364
              tunnel: [w401] -> w363
              tunnel: [w390] -> w356
              tunnel: w352 -> [w389]
              tunnel: w351 -> [w388]
              tunnel: [w389] -> w350
              tunnel: [w388] -> w349
              tunnel: [w423] -> w377
              tunnel: [w440] -> w376
              tunnel: [w439] -> w375
              tunnel: [w438] -> w374
              tunnel: [w431] -> w373
              tunnel: w368 -> [w437]
              tunnel: w367 -> [w436]
              tunnel: w366 -> [w435]
              tunnel: w365 -> [w434]
              tunnel: w364 -> [w433]
              tunnel: w363 -> [w432]
              tunnel: w356 -> [w429]
              tunnel: [w428] -> w355
              tunnel: w350 -> [w427]
              tunnel: w349 -> [w426]
              tunnel: [w424] -> w348
              tunnel: w377 -> [w591]
              tunnel: w376 -> [w582]
              tunnel: w375 -> [w581]
              tunnel: w374 -> [w607]
              tunnel: [w637] -> w360
              tunnel: w373 -> [w639]
              tunnel: [w623] -> w370
              tunnel: [w624] -> w372
              tunnel: [w625] -> w371
              tunnel: w355 -> [w601]
              tunnel: w348 -> [w592]
              tunnel: [w592] -> w346
              tunnel: [w591] -> w345
              frame #0 {
                n178 = local read "Offset_rueda WS 1"() -> (w381:fxp<+/-,24,-4>)
                n179 = local read "Offset_rueda WS 2"() -> (w382:fxp<+/-,24,-4>)
                n180 = local read "Frecuencia de muestreo (Hz)"() -> (w399:dbl)
                n181 = local read "Canal cero WS1?"() -> (w392:bool)
                n182 = local read "Escaneos de la FIFO por canal"() -> (w387:u32)
                n183 = local read "Count(mSec)"() -> (w391:u32)
                n184 = local read "Frecuencia de muestreo y módulo CRIO"() -> (w394:T3)
                n185 = local read "Canal cero WS2"() -> (w380:bool)
                n186 = local read "Digital?"() -> (w393:bool)
                n187 = local read "RFID LR6 on?"() -> (w383:bool)
                n188 = xnode "Read/Write Control"("FPGA VI Reference In"=w408, "error in"=w407, "Data Rate"=w394, "Digital?"=w393, "Canal cero WS1?"=w392, "Count(mSec)"=w391, "Offset_WS1"=w381, "Offset_WS2"=w382, "Canal cero WS2?"=w380) -> ("FPGA VI Reference Out"=w398:refnum<k20>, "error out"=w397:errorcluster)
                n189 = case shown="False" w383 {
                  tunnel: [errorcluster {"status"=FALSE, "code"=0, "source"=""} ("error out") w413] -> w390
                  frame False {
                  }
                  frame True {
                    n190 = local read "RFID_LR6_Error"() -> (w414:errorcluster)
                    n191 = call "LH6HD.vi"("error in (no error)"=w414, "Action"=enum16{"Init", "Start", "Read", "Stop", "Exit"}."Start") -> ("error out"=w413:errorcluster)  [unwired: 8 in, 1 out]
                  }
                }
                n192 = Add(x="Nº inductivos", y="Nº de acelerómetros") -> (x+y=w385:i32)
                n193 = call "DMACalc.vi"("Number of Channels"=w385, "Number of Samples"=w387, "Rate (Hz)"=w399) -> ("Block Size"=w403:u32, "Time to Acquire Block (ms)"=w404:i32, "Host Buffer Size"=w409:u32)  [unwired: 6 in]
                n194 = call "Pathhorafech(SubVI)_varios.vi"("Folder path"=path "c:/Trenes", "Nº de acelerómetros"="Nº de acelerómetros", "Nº inductivos"="Nº inductivos") -> ("Acel_Paths"=w395:path[])  [unwired: 1 in, 1 out]
                "Nombre de archivo" <- w395
                n195 = for {
                  tunnel: w395 -> [w418] mode=indexing
                  tunnel: [w417] -> w402 mode=indexing
                  tunnel: [w416] -> w401
                  n196 = Open/Create/Replace File(file path (use dialog)=w418, operation (0:open)=T6."replace or create", access (0:read/write)=enum16{"read/write", "read-only", "write-only"}."read/write", disable buffering (F)=TRUE) -> (refnum out=w417:refnum<file>, error out=w416:errorcluster)  [unwired: 1 in, 2 out]
                }
                n197 = xnode "Invoke Method"("FPGA VI Reference In"=w398, "error in"=w397, "Requested Depth"=w409) -> ("FPGA VI Reference Out"=w411:refnum<k20>, "error out"=w410:errorcluster)  [unwired: 1 out]
                n198 = Get Date/Time In Seconds() -> (seconds since 1Jan1904=→"Inicio pasada":timestamp)
                n199 = xnode "Invoke Method"("FPGA VI Reference In"=w411, "error in"=w410) -> ("FPGA VI Reference Out"=w406:refnum<k20>, "error out"=w405:errorcluster)
              }
              frame #1 {
                n200 = while "Data Acquisition" {
                  tunnel: w437 -> [w492]
                  shift-right: [w517] -> _
                  shift-left: u32 0 ("t") -> [w513]
                  tunnel: w435 -> [w518]
                  tunnel: w434 -> [w516]
                  shift-right: [w519] -> w439
                  shift-left: w436 -> [w510]
                  tunnel: [w514] -> w440
                  tunnel: w433 -> [w496]
                  tunnel: [w497] -> w438
                  shift-right: [w495] -> w431
                  shift-left: w432 -> [w506]
                  i -> [w491]
                  stop <- w515 stop-if-true
                  # "Detector de presencia"
                  # "Mide el tiempo de paso del tren y con ello se puede calcular\nla velocidad la unidad"
                  n201 = xnode "Invoke Method"("FPGA VI Reference In"=w492, "error in"=w510, "Number of Elements"=w513, "Timeout (ms)"=0) -> ("FPGA VI Reference Out"=w488:refnum<k20>, "error out"=w494:errorcluster, "Data"=w509:fxp<+/-,24,4>[], "Elements Remaining"=w511:u32)
                  n202 = case "Data Ready" shown="Default" w513 {
                    tunnel: w518 -> [w541 _]
                    tunnel: [w540 u32 0 ("t")] -> w517
                    tunnel: w516 -> [w542 _]
                    tunnel: w511 -> [w539 _]
                    tunnel: w509 -> [_ w564]
                    tunnel: w506 -> [w538 w563]
                    tunnel: [w538 w565] -> w495
                    tunnel: w496 -> [w537 w562]
                    tunnel: [w537 w561] -> w497
                    frame 0 {
                      # "En este caso se compara los elementos que quedan\nen la FIFO del controlador con el tamaño dell bloque\nque aparece en el panel frontal. Si el número de \nelementos en la FIFO es mayor o igual que el tamaño\n del bloque se pasa al siguiente caso y se guardan \nlos datos en un archivo. El reloj que aparece es una\nespera para no consumir recursos."
                      n203 = Greater Or Equal?(x=w539, y=w542) -> (x >= y?=w543:bool)
                      n204 = case shown="False" w543 {
                        tunnel: [u32 0 ("Block Size") w547] -> w540
                        tunnel: [w546 0 ("t")] -> w544
                        tunnel: w541 -> [w546 _]
                        tunnel: w542 -> [_ w547]
                        frame False {
                        }
                        frame True {
                        }
                      }
                      n205 = call "WaitMinTimeBetweenCall.vi"("Minimum ms between calls"=w544) -> ()  [unwired: 2 in]
                    }
                    frame Default {
                      n206 = To Single Precision Float(number=w564) -> (single precision float=w551:sgl[])
                      n207 = Decimate 1D Array(w551) -> (w557:sgl[], w560:sgl[], w559:sgl[], w558:sgl[], w556:sgl[], w555:sgl[], w554:sgl[], w553:sgl[], w552:sgl[], w549:sgl[])
                      n208 = Build Array(w557, w560, w559, w558, w556, w555, w554, w553, w552, w549) -> (w550:sgl[][])
                      n209 = for {
                        tunnel: T7."little-endian" ("byte order (0:big-endian, network order)") -> [w574]
                        shift-right: [w568] -> w565
                        shift-left: w563 -> [w569]
                        tunnel: w550 -> [w572] mode=indexing
                        tunnel: w562 -> [w571] mode=indexing
                        tunnel: [w570] -> w561 mode=indexing
                        n210 = Write to Binary File(file (use dialog)=w571, data=w572, error in=w569, 5:FALSE ("prepend array or string size? (T)"), 9:w574) -> (refnum out=w570:refnum<file>, error out=w568:errorcluster)  [unwired: 2 out]
                      }
                    }
                  }
                  n211 = xnode "Read/Write Control"("FPGA VI Reference In"=w488, "error in"=w494) -> ("FPGA VI Reference Out"=w508:refnum<k20>, "error out"=w507:errorcluster, "Parar"=w484:bool, "Nº Ruedas 1"=→"Nº Ruedas 1":i32, "NºRuedas 2"=→"NºRuedas 2":i32)
                  "Parar" <- w484
                  n212 = case shown="False" w484 {
                    tunnel: [w523 w532] -> w485
                    tunnel: [w525 0.0] -> w500
                    frame False {
                      n213 = local read "Inicio pasada"() -> (w528:timestamp)
                      n214 = Get Date/Time In Seconds() -> (seconds since 1Jan1904=w527:timestamp)
                      n215 = To Double Precision Float(number=w527) -> (double precision float=w526:dbl)
                      n216 = To Double Precision Float(number=w528) -> (double precision float=w529:dbl)
                      n217 = Subtract(x=w526, y=w529) -> (x-y=w525:dbl)
                      "Tiempo de paso (s)" <- w525
                      n218 = local write "Tiempo"(w526) -> ()
                      n219 = local read "Boton Adquirir?"() -> (w520:bool)
                      n220 = Greater?(x=w525, y="Tiempo de adquisicion") -> (0:w522:bool)
                      n221 = Select(t=w522, s=w520, f=FALSE) -> (s? t:f=w523:bool)
                    }
                    frame True {
                      n222 = local read "Tiempo"() -> (w536:dbl)
                      n223 = local read "Tiempo extra al detector de paso (s)"() -> (w531:dbl)
                      n224 = Get Date/Time In Seconds() -> (seconds since 1Jan1904=w533:timestamp)
                      n225 = To Double Precision Float(number=w533) -> (double precision float=w534:dbl)
                      n226 = Subtract(x=w534, y=w536) -> (x-y=w535:dbl)
                      "Tiempo extra de adquisición (s)" <- w535
                      n227 = Greater?(x=w535, y=w531) -> (0:w532:bool)
                    }
                  }
                  "Fin" <- w485
                  n228 = local read "Timeout ruedas"() -> (w483:dbl)
                  n229 = xnode ("CheckLate")("FPGA VI Reference In"=w508, "error in"=w507) -> ("FPGA VI Reference Out"=w490:refnum<k20>, "error out"=w503:errorcluster, "Buffer Underflow"=→"Buffer Underflow":bool, "Buffer Overflow"=w493:bool)
                  "Buffer Overflow" <- w493
                  n230 = Greater?(x=w500, y=w483) -> (0:w498:bool)
                  "Timeout ruedas" <- w498
                  n231 = call "ErrorOverFlow.vi"("Buffer Overflow"=w493) -> ("error out"=w501:errorcluster)
                  n232 = call "ErrorUnderFlow.vi"() -> ("error out"=w502:errorcluster)  [unwired: 1 in]
                  n233 = Merge Errors(w503, w502, w501) -> (w489:errorcluster)
                  n234 = Unbundle By Name(w495) -> ("status"=w499:bool)
                  n235 = Unbundle By Name(w489) -> ("status"=w505:bool)
                  n236 = Compound Arithmetic op=OR(w505, w485, w498, w499) -> (w515:bool)
                  "result" <- w515
                  n237 = case "Flush" shown="True" w515 {
                    tunnel: [w575 w580] -> w519
                    tunnel: [w576 w579] -> w514
                    tunnel: w490 -> [w576 w578]
                    tunnel: w489 -> [w575 w577]
                    frame False {
                    }
                    frame True {
                      n238 = xnode "Invoke Method"("FPGA VI Reference In"=w578, "error in"=w577) -> ("FPGA VI Reference Out"=w579:refnum<k20>, "error out"=w580:errorcluster)
                    }
                  }
                  "Block Size" <- w516
                  "Time to Acquire Block (ms)" <- w518
                  "Numeric 3" <- w491
                }
                n239 = call <vilib>:"Watchdog Whack.vi"("error in (no error)"=w426, "reset watchdog after expire? (F)"=TRUE, "watchdogID in"=w427) -> ("error out"=w423:errorcluster, "watchdogID out"=w424:u64)  [unwired: 2 in, 1 out]
                n240 = local read "RFID LR6 on?"() -> (w422:bool)
                n241 = case shown="True" w422 {
                  tunnel: w429 -> [w441 w447]
                  tunnel: [w441 w446] -> w428
                  frame False {
                  }
                  frame True {
                    n242 = while {
                      shift-right: [w454] -> w446
                      shift-left: w447 -> [w455]
                      shift-right: [w453] -> w444
                      shift-left: string[] [] -> [w452]
                      shift-right: [w448] -> w442
                      shift-left: i32[] [] -> [w449]
                      i -> [w450]
                      stop <- w451 stop-if-true
                      n243 = case shown="No Error" w455 {
                        selector: w455 -> [w466 _]
                        tunnel: [w465 w481] -> w454
                        tunnel: [w461 string[] []] -> w453
                        tunnel: w452 -> [w460 _]
                        tunnel: w450 -> [w459 _]
                        tunnel: w449 -> [w458 _]
                        tunnel: [w457 i32[] []] -> w448
                        frame No Error {
                          n244 = call "LH6HD.vi"("error in (no error)"=w466, "Action"=enum16{"Init", "Start", "Read", "Stop", "Exit"}."Read") -> ("error out"=w465:errorcluster, "Tag"=w462:string)  [unwired: 8 in]
                          n245 = Not Equal?(x="", y=w462) -> (x != y?=w463:bool)
                          n246 = case shown="False" w463 {
                            tunnel: w462 -> [_ w475]
                            tunnel: [w469 w474] -> w461
                            tunnel: w460 -> [w469 w473]
                            tunnel: w459 -> [_ w470]
                            tunnel: w458 -> [w468 w472]
                            tunnel: [w468 w471] -> w457
                            frame False {
                            }
                            frame True {
                              n247 = Build Array (concatenate)(w473, w475) -> (w474:string[])
                              n248 = Build Array (concatenate)(w472, w470) -> (w471:i32[])
                            }
                          }
                        }
                        frame Error {
                          n249 = local read "LR6 IP address"() -> (w478:string)
                          n250 = local read "DeviceAddress"() -> (w476:u8)
                          n251 = local read "Port LR6"() -> (w479:u16)
                          n252 = call "LH6HD.vi"("DeviceAddress"=w476, "Reader Port"=w479, "IP Address"=w478, "Action"=enum16{"Init", "Start", "Read", "Stop", "Exit"}."Init") -> ("error out"=w481:errorcluster)  [unwired: 6 in, 1 out]
                        }
                      }
                      n253 = Wait Until Next ms Multiple(millisecond multiple=u32 500) -> ()  [unwired: 1 out]
                      n254 = local read "result"() -> (w451:bool)
                      "it-LR6" <- w450
                    }
                    "TAGs LR6" <- w444
                    "it-read-LR6" <- w442
                  }
                }
              }
              frame #2 {
                n255 = local read "RFID LR6 on?"() -> (w583:bool)
                n256 = Array Size(array=w607) -> (size(s)=w605:i32)
                n257 = local read "TAGs LR6"() -> (w594:string[])
                n258 = local read "timeout ms (60000)"() -> (w590:i32)
                n259 = local read "bytes to read"() -> (w589:i32)
                n260 = local read "RFID NEM on?"() -> (w588:bool)
                n261 = Decrement(x=w605) -> (x-1=w606:i32)
                n262 = local read "Puerto RFID"() -> (w622:u16)
                n263 = case shown="False" w583 {
                  tunnel: w601 -> [w647 w649]
                  tunnel: [w647 w648] -> w600
                  frame False {
                  }
                  frame True {
                    n264 = call "LH6HD.vi"("error in (no error)"=w649, "Action"=enum16{"Init", "Start", "Read", "Stop", "Exit"}."Stop") -> ("error out"=w648:errorcluster)  [unwired: 8 in, 1 out]
                  }
                }
                n265 = local read "RFID_Error"() -> (w633:errorcluster)
                n266 = local read "IP RFID"() -> (w604:string)
                n267 = local read "RFID_ID"() -> (w632:refnum<k5>)
                n268 = Index Array(array=w607, index=w606) -> (element=w615:refnum<file>)
                n269 = local write "result"(FALSE ("result")) -> ()
                n270 = case shown="True" w588 {
                  tunnel: [_ w662] -> w634
                  tunnel: w633 -> [w652 w661]
                  tunnel: w632 -> [w651 w660]
                  tunnel: [w651 w659] -> w631
                  tunnel: [w652 w658] -> w626
                  tunnel: w622 -> [_ w657]
                  tunnel: w604 -> [_ w656]
                  tunnel: [_ w655] -> w587
                  tunnel: w590 -> [_ w654]
                  tunnel: w589 -> [_ w653]
                  frame False {
                  }
                  frame True {
                    n271 = call "RFID_28_03_12.vi"("BYTES TO READ"=w653, "TIMEOUT"=w654, "RFID_Error"=w661, "Puerto RFID"=w657, "IP RFID"=w656, "RFID ID"=w660) -> ("RFID Error"=w658:errorcluster, "connection ID out"=w659:refnum<k5>, "TAGs HEX"=w655:string[], "Unidad"=w662:u32)  [unwired: 1 in]
                  }
                }
                n272 = local write "RFID_LR6_Error"(w600) -> ()
                n273 = for {
                  tunnel: w594 -> [w665] mode=indexing
                  tunnel: [w663] -> w593 mode=indexing
                  n274 = Search and Replace String(input string=w665, search string="00") -> (result string=w663:string)  [unwired: 6 in, 3 out]
                }
                n275 = Delete From Array(array=w587, length=1, index=0) -> (array with subset deleted=w584:string[])  [unwired: 1 out]
                "TAGs HEX" <- w584
                n276 = xnode "Read/Write Control"("FPGA VI Reference In"=w582, "error in"=w581) -> ("FPGA VI Reference Out"=w636:refnum<k20>, "error out"=w635:errorcluster, "Chassis Temperature"=w645:i16)
                n277 = Index Array(array=w584) -> (element=w599:string)  [unwired: 1 in]
                n278 = Not Equal?(x=w599, y="" ("delimiter (\\t)")) -> (x != y?=w597:bool)
                "Plataformas?" <- w597
                n279 = case shown="True" w597 {
                  tunnel: w593 -> [w666 w667]
                  tunnel: [w666 w669] -> w602
                  tunnel: w584 -> [_ w668]
                  frame False {
                  }
                  frame True {
                    n280 = call "Union_TAGs_RFIDs.vi"("TAGs LR6"=w667, "TAGs HEX"=w668) -> ("TAGs"=w669:string[])
                  }
                }
                "TAGs" <- w602
                n281 = Divide(x=w645, y=4.0) -> (x/y=w646:dbl)
                "Temperatura (ºC)" <- w646
                n282 = local read "Tiempo de paso (s)"() -> (w629:dbl)
                n283 = local read "Nombre de archivo"() -> (w614:path[])
                n284 = Multiply(x=w629, y=1000.0) -> (x*y=w627:dbl)
                n285 = for {
                  shift-right: [w675] -> w620
                  shift-left: string[] [] -> [w674]
                  tunnel: w602 -> [w673] mode=indexing
                  n286 = Insert Into Array(array=w674, new element=w673) -> (w675:string[])  [unwired: 1 in]
                }
                n287 = Build Array(w646, w627, w634) -> (w640:dbl[])
                n288 = local write "RFID_ID"(w631) -> ()
                n289 = local write "RFID_Error"(w626) -> ()
                n290 = Delete From Array(array=w614) -> (deleted portion=w613:path)  [unwired: 2 in, 1 out]
                n291 = To Single Precision Float(number=w640) -> (single precision float=w643:sgl[])
                n292 = xnode "Read/Write Control"("FPGA VI Reference In"=w636, "error in"=w635, "Stop"=TRUE ("stop")) -> ("FPGA VI Reference Out"=w617:refnum<k20>, "error out"=w616:errorcluster)
                n293 = Path To String(path=w613) -> (string=w619:string)
                n294 = Write to Binary File(file (use dialog)=w615, data=w643, error in=w639, 5:FALSE ("prepend array or string size? (T)"), 9:T7."little-endian" ("byte order (0:big-endian, network order)")) -> (error out=w612:errorcluster)  [unwired: 3 out]
                n295 = local read "Timeout ruedas"() -> (w630:bool)
                n296 = Build Array (concatenate)(w619, w620) -> (w595:string[])
                n297 = local read "TAGS leidos"() -> (w608:path)
                n298 = for {
                  shift-right: [w672] -> w623
                  shift-left: w612 -> [w671]
                  tunnel: w607 -> [w670] mode=indexing
                  n299 = Close File(refnum=w670, error in=w671) -> (error out=w672:errorcluster)  [unwired: 1 out]
                }
                n300 = xnode "Invoke Method"("FPGA VI Reference In"=w617, "error in"=w616) -> ("FPGA VI Reference Out"=w625:refnum<k20>, "error out"=w624:errorcluster)
                n301 = call-poly <vilib>:"Write Delimited Spreadsheet.vi"("file path (dialog if empty)"=w608, "1D data"=w595, "append to file? (F)"=FALSE ("transpose? (no:F)"), "transpose? (F)"=TRUE ("append to file? (new file:F)"), "delimiter (\\t)"=";" ("delimiter (\\t)")) -> ()  [unwired: 9 in, 2 out]
                n302 = Select(t="TEST", s=w630, f="Procesado") -> (s? t:f=w637:string)
              }
            }
            n303 = call <vilib>:"Watchdog Clear.vi"("error in (no error)"=w345, "watchdogID in"=w346) -> ("error out"=w347:errorcluster)  [unwired: 5 in]
            n304 = Unbundle By Name(w372) -> ("status"=w361:bool)
            n305 = Unbundle By Name(w370) -> ("status"=w362:bool)
            n306 = Merge Errors(w370, w347) -> (w369:errorcluster)
            n307 = Compound Arithmetic op=OR(w361, w362) -> (w359:bool)
            n308 = Select(t="TEST", s=w359, f=w360) -> (s? t:f=w357:string)
          }
          frame "Procesado" {
            n309 = local read "Watchdog config"() -> (w682:T1)
            n310 = call <vilib>:"Watchdog Configure.vi"("error in (no error)"=w685, "expiration actions"=w682, "timeout (1 sec)"=300.0) -> ("error out"=w684:errorcluster, "watchdogID"=w681:u64)  [unwired: 3 in, 2 out]
            n311 = flat-sequence {
              tunnel: w684 -> [w707]
              tunnel: [w710] -> w687
              tunnel: w681 -> [w702]
              tunnel: [w701] -> w680
              tunnel: [w700] -> w679
              tunnel: [w906] -> w697
              tunnel: w687 -> [w906]
              tunnel: [w899] -> w678
              tunnel: w680 -> [w899]
              tunnel: [w898] -> w677
              tunnel: w679 -> [w898]
              frame #0 {
                n312 = flat-sequence {
                  tunnel: [w782] -> w709
                  tunnel: [w766] -> w708
                  tunnel: w707 -> [w731]
                  tunnel: [w769] -> w706
                  tunnel: [w756] -> w703
                  tunnel: [w768] -> w705
                  tunnel: [w755] -> w704
                  tunnel: w702 -> [w732]
                  tunnel: [w729] -> w701
                  tunnel: [w728] -> _
                  tunnel: [w728] -> w700
                  frame #0 {
                    # "No es necesario leer el segundo archivo"
                    # "Estos indicadores sirven para controlar que no se sature la memoria"
                    # "Distancia de\nla unidad"
                    n313 = disable-structure shown="Enabled" {
                      disable-tunnel: [w785 "Array"] -> w722
                      frame Disabled {
                        n314 = local read "Nombre de archivo"() -> (w785:path[])
                      }
                      frame Enabled {
                      }
                    }
                    n315 = local read "Tabla_flota"() -> (w765:string[][])
                    n316 = call <vilib>:"Watchdog Whack.vi"("error in (no error)"=w731, "reset watchdog after expire? (F)"=TRUE, "watchdogID in"=w732) -> ("error out"=w728:errorcluster, "watchdogID out"=w729:u64)  [unwired: 2 in, 1 out]
                    n317 = local read "TAGs"() -> (w759:string[])
                    n318 = call "Series_ejes_flota.vi"("Tabla_flota"=w765, "Tags"=w759) -> ("Nº Ejes"=w721:i32[], "Series del convoy"=w758:string[])  [unwired: 2 in, 1 out]
                    "Nº Ejes" <- w721
                    n319 = local read "Puntos medios de las ventanas"() -> (w767:dbl[][])
                    n320 = Array Size(array=w722) -> (size(s)=w775:i32)
                    n321 = Add Array Elements(numeric array=w721) -> (sum=w727:i32)
                    "Ejes_convoy" <- w727
                    n322 = Subtract(x=w775, y=2 ("length")) -> (x-y=w777:i32)
                    n323 = Array Size(array=w758) -> (size(s)=→"Nº UTs":i32)
                    n324 = Delete From Array(array=w722, length=2, index=w777) -> (deleted portion=w745:path[], array with subset deleted=w768:path[])
                    n325 = Index Array(array=w745) -> (element #1=w723:path, element #2=w724:path)  [unwired: 2 in]
                    n326 = Read from Binary File(5:sgl 0.0, 9:T7."little-endian" ("byte order (0:big-endian, network order)"), 10:-1 ("count (1)"), 11:w724) -> (0:w773:errorcluster, 2:w747:sgl[], 3:w774:refnum<file>)  [unwired: 1 in, 2 out]
                    n327 = local read "Series_flota"() -> (w764:string[])
                    n328 = Close File(refnum=w774, error in=w773) -> (error out=w769:errorcluster)  [unwired: 1 out]
                    n329 = Read from Binary File(5:sgl 0.0, 9:T7."little-endian" ("byte order (0:big-endian, network order)"), 10:-1 ("count (1)"), 11:w723) -> (0:w743:errorcluster, 2:w735:sgl[], 3:w744:refnum<file>)  [unwired: 1 in, 2 out]
                    n330 = Array Size(array=w747) -> (size(s)=w763:i32)
                    n331 = Close File(refnum=w744, error in=w743) -> ()  [unwired: 2 out]
                    n332 = Subtract(x=w763, y=3 ("length")) -> (x-y=w761:i32)
                    n333 = Array Size(array=w735) -> (size(s)=w739:i32)
                    n334 = Delete From Array(array=w747, length=3, index=w761) -> (deleted portion=→"deleted portion":sgl[], array with subset deleted=w712:sgl[])
                    n335 = call "Distancias_ejes_convoy.vi"("Series_flota1"=w758, "Ejes_UT"=w721, "Puntos medios de las ventanas"=w767, "Series_flota"=w764) -> ("Distancias_entre_ejes_convoy"=w766:dbl[])  [unwired: 1 in]
                    n336 = Subtract(x=w739, y=3 ("length")) -> (x-y=w737:i32)
                    n337 = call "Puntos medio de pulso.vi"("DI Inductivo"=w712) -> ("Puntos"=w782:sgl[], "Número de ejes"=w748:i32)  [unwired: 1 in]
                    "Número de ejes detectados" <- w748
                    n338 = Delete From Array(array=w735, length=3, index=w737) -> (deleted portion=→"deleted portion 2":sgl[], array with subset deleted=w734:sgl[])
                    n339 = Decrement(x=w748) -> (x-1=w781:i32)
                    n340 = local read "Tiempo de paso (s)"() -> (w780:dbl)
                    n341 = Build Array(w712, w734) -> (→"Waveform Graph":sgl[][])
                    n342 = local read "TAGs"() -> (w754:string[])
                    n343 = local read "it-LR6"() -> (w751:i32)
                    n344 = local read "it-read-LR6"() -> (w752:i32[])
                    n345 = local read "TAGs LR6"() -> (w753:string[])
                    n346 = local read "Plataformas?"() -> (w750:bool)
                    n347 = call "Calculo_Velocidad.vi"("Tiempo de paso (s)"=w780, "Ejes"=w781, "Puntos iniciales de las ventanas"=w766) -> ("V (m/s)"=→"V (m/s)":dbl, "Longitud de la unidad"=→"Longitud de la unidad":dbl)
                    n348 = call "TAGs_AURAwheel.vi"("Nº Ejes"=w721, "TAGs"=w754, "Ejes_convoy"=w727, "it-LR6"=w751, "TAGs LR6"=w753, "it-read-LR6"=w752, "Plataformas?"=w750) -> ("TAGS_AURA"=→"TAGs_AURAwheel":string[][])  [unwired: 1 in]
                    n349 = Equal?(x=w712, y=0.0) -> (x = y?=w716:bool[])
                    n350 = Equal?(x=w712, y=1.0) -> (x = y?=w717:bool[])
                    n351 = Or(x=w716, y=w717) -> (x .or. y?=w713:bool[])
                    n352 = Search 1D Array(1D array=w713, element=FALSE) -> (index of element=w719:i32)  [unwired: 1 in]
                    n353 = Get Volume Info(11:path "c:/" ("path")) -> (1:→"Disco Duro Disponible (bytes)":i64)  [unwired: 1 in, 5 out]
                    n354 = Equal?(x=w727, y=w748) -> (x = y?=w755:bool)
                    n355 = Equal?(x=w719, y=-1) -> (x = y?=w711:bool)
                    "Problema WS" <- w711
                    n356 = And(x=w755, y=w711) -> (x .and. y?=w756:bool)
                  }
                }
                n357 = case shown="True" w703 {
                  tunnel: w706 -> [w789 w820]
                  tunnel: [w789 w819] -> w710
                  tunnel: w709 -> [_ w824]
                  tunnel: w708 -> [_ w822]
                  tunnel: w705 -> [_ w823]
                  tunnel: w704 -> [w787 _]
                  frame False {
                    n358 = local read "Nombre de archivo"() -> (w788:path[])
                    n359 = for {
                      tunnel: w788 -> [w791] mode=indexing
                      tunnel: w787 -> [w790]
                      n360 = flat-sequence {
                        tunnel: w791 -> [w801]
                        tunnel: [w801] -> w794
                        tunnel: [w800] -> w793
                        tunnel: w790 -> [w799]
                        tunnel: w794 -> [w808]
                        tunnel: [w807] -> w792
                        tunnel: w793 -> [w807]
                        tunnel: w792 -> [w810]
                        frame #0 {
                          w800 = path "c:/Est_Adq.csv" ("file path (use dialog)")
                          n361 = Path To String(path=w801) -> (string=w802:string)
                          n362 = Select(t="Nº Ejes detectados WS diferente a Nº Ejes TAGs" ("delimiter (\\t)"), s=w799, f="La señal del inductivo no es digital" ("delimiter (\\t)")) -> (s? t:f=w796:string)
                          n363 = Build Array(w802, w796) -> (w795:string[])
                          n364 = call-poly <vilib>:"Write Delimited Spreadsheet.vi"("file path (dialog if empty)"=w800, "1D data"=w795, "append to file? (F)"=FALSE ("transpose? (no:F)"), "transpose? (F)"=TRUE ("append to file? (new file:F)"), "delimiter (\\t)"=";" ("delimiter (\\t)")) -> ()  [unwired: 9 in, 2 out]
                        }
                        frame #1 {
                          n365 = local read "Borrar archivos\nadquisicion con error"() -> (w806:bool)
                          n366 = case shown="True" w806 {
                            tunnel: w808 -> [_ w809]
                            frame False {
                            }
                            frame True {
                              n367 = Delete(path (use dialog)=w809) -> ()  [unwired: 1 in, 6 out]
                            }
                          }
                        }
                        frame #2 {
                          n368 = File/Directory Info(path=w810) -> (size=w813:i64)  [unwired: 1 in, 6 out]
                          n369 = Greater?(x=w813, y=i64 1000000) -> (0:w811:bool)
                          n370 = case shown="True" w811 {
                            tunnel: w810 -> [_ w814]
                            frame False {
                            }
                            frame True {
                              n371 = Delete(path (use dialog)=w814) -> ()  [unwired: 4 in, 3 out]
                            }
                          }
                        }
                      }
                    }
                  }
                  frame True {
                    n372 = flat-sequence {
                      tunnel: w824 -> [w892]
                      tunnel: w823 -> [w889]
                      tunnel: w822 -> [w893]
                      tunnel: [w887] -> w821
                      frame #0 {
                        # "SALIDA \n\nMáximos por rueda inductivo"
                        # "8 acelerómetros"
                        # "Velocidad"
                        n373 = local read "Frecuencia de muestreo (Hz)"() -> (w891:dbl)
                        n374 = local read "Distancia de acelerómetros"() -> (w879:dbl[])
                        n375 = local read "Parámetros acelerómetros"() -> (w886:dbl[])
                        n376 = local read "Número de ejes detectados"() -> (w885:i32)
                        n377 = local read "Distancias generales"() -> (w884:dbl[])
                        n378 = local read "dt RMS"() -> (w890:dbl)
                        n379 = local read "Direccion 0?"() -> (w876:bool)
                        n380 = Index Array(array=w884, index=1) -> (element=w882:dbl)
                        n381 = Select(t=0.0, s=w876, f=w882) -> (s? t:f=w880:dbl)
                        n382 = Subtract(x=w880, y=w879) -> (x-y=w878:dbl[])
                        n383 = Absolute Value(x=w878) -> (abs(x)=w877:dbl[])
                        n384 = call "Procesado_aRMS_BIdirecc.vi"("Paths_canales_aRMS"=w889, "Ejes Procesados"=w885, "Distancias\nacelerometros"=w877, "Distancias generales (m)"=w884, "Distancias centrales de las ruedas\n               configuración (m)"=w893, "Frecuencia de muestreo"=w891, "Parámetros acelerómetros"=w886, "dt RMS 2"=w890, "Puntos"=w892) -> ("Max RMS Ruedas"=w888:dbl[][])  [unwired: 2 in]
                        n385 = Transpose 2D Array(2D array=w888) -> (transposed array=w887:dbl[][])
                        "Max RMS Ruedas" <- w887
                      }
                    }
                    n386 = local read "Use Aura?"() -> (w818:bool)
                    n387 = local read "TAGs_AURAwheel"() -> (w816:string[][])
                    n388 = local read "Nº Ejes"() -> (w815:i32[])
                    n389 = for {
                      tunnel: w818 -> [w829]
                      tunnel: [w828] -> w817 mode=indexing
                      tunnel: w816 -> [w827] mode=indexing
                      shift-right: [w826] -> _
                      shift-left: w821 -> [w830]
                      tunnel: w815 -> [w825] mode=indexing
                      # "dev.api.aurawheel.com"
                      n390 = case shown="True" w829 {
                        tunnel: w830 -> [w831 w841]
                        tunnel: [errorcluster {"status"=FALSE, "code"=0, "source"=""} ("error out") w846] -> w828
                        tunnel: w827 -> [_ w842]
                        tunnel: [w831 w840] -> w826
                        tunnel: w825 -> [_ w838]
                        frame False {
                        }
                        frame True {
                          w850 = cluster{"status":string} {"status"=""}
                          n391 = local read "Parametros AuraWheel"() -> (w875:string[])
                          n392 = Delete From Array(array=w841, length=w838, index (row)=0) -> (deleted portion=w837:dbl[][], array with subset deleted=w840:dbl[][])  [unwired: 1 in]
                          n393 = Get Date/Time In Seconds() -> (seconds since 1Jan1904=w871:timestamp)
                          n394 = Format Date/Time String(time format string (%c)="%H:%M:%S%3u", seconds (now)=w871) -> (date/time string=w869:string)  [unwired: 1 in]
                          n395 = Get Date/Time In Seconds() -> (seconds since 1Jan1904=w845:timestamp)
                          n396 = Scan From String(format string="%d:%d:%f", input string=w869) -> (output 1=w866:i32, output 2=w865:i32, output 3=w863:dbl)  [unwired: 5 in, 3 out]
                          n397 = local read "Temperatura (ºC)"() -> (w843:dbl)
                          n398 = local read "V (m/s)"() -> (w833:dbl)
                          n399 = Multiply(x=w863, y=1000.0) -> (x*y=w859:dbl)
                          n400 = call "Time_to_ms.vi"("seconds since 1Jan1904"=w845) -> ("Numeric"=w844:dbl)  [unwired: 1 in]
                          n401 = Multiply(x=w865, y=60000) -> (x*y=w860:i32)
                          n402 = Multiply(x=3600000, y=w866) -> (x*y=w861:i32)
                          n403 = Index Array(array=w875) -> (element #1=w836:string, element #2=w835:string, element #3=w834:string)  [unwired: 3 in]
                          n404 = call "aw_WRDCluster_8acel.vi"("Array TAGs"=w842, "Max RMS Ruedas"=w837, "TimeStamp"=w844, "p_sp"=w833, "p_tp"=w843) -> ("JSON cluster"=w872:T9)  [unwired: 1 in]
                          n405 = Compound Arithmetic op=ADD(w861, w860, w859) -> (w858:dbl)
                          n406 = To Variant(anything=w872) -> (Variant=w855:variant)
                          n407 = To Unsigned Long Integer(number=w858) -> (unsigned 32bit integer=w857:u32)
                          n408 = call "gjson_Create.vi"("JSON Object in"=w855) -> ("error out"=w853:errorcluster, "JSON String Out"=w854:string)  [unwired: 9 in]
                          n409 = Number To Decimal String(number=w857) -> (decimal integer string=w856:string)  [unwired: 1 in]
                          n410 = To Variant(anything=w850) -> (Variant=w849:variant)
                          n411 = call "aw_SendData.vi"("pwd"=w836, "x-nem-datetime"=w856, "User"=w835, "error in"=w853, "JSON Object"=w854, "URL"=w834) -> ("error out"=w851:errorcluster, "Response JSON"=w852:string, "Response headers"=→"Response headers":string)  [unwired: 3 in]
                          n412 = call "gjson_Parse.vi"("error in"=w851, "JSON String In"=w852, "JSON Cluster"=w849) -> ("error out"=w847:errorcluster, "JSON Cluster Out"=w848:variant)  [unwired: 7 in]
                          n413 = Variant To Data(error in=w847, type=w850, Variant=w848) -> (data=→"data":cluster{"status":string}, error out=w846:errorcluster)
                          "error AURA" <- w846
                        }
                      }
                    }
                    n414 = Merge Errors(w817, w820) -> (w819:errorcluster)
                  }
                }
              }
              frame #1 {
                n415 = local read "Bytes libre despues de borrar"() -> (w895:u32)
                n416 = local read "Bytes min libre"() -> (w896:u32)
                n417 = local read "Max archivos"() -> (w897:u32)
                n418 = local read "TAGS leidos"() -> (w902:path)
                n419 = local read "Nombre de archivo"() -> (w900:path[])
                n420 = File/Directory Info(path=w902) -> (size=w905:i64)  [unwired: 1 in, 6 out]
                n421 = local read "Path TEST"() -> (w901:path)
                n422 = Greater?(x=w905, y=i64 1000000) -> (0:w903:bool)
                n423 = case shown="True" w903 {
                  tunnel: w902 -> [_ w907]
                  frame False {
                  }
                  frame True {
                    n424 = Delete(path (use dialog)=w907) -> ()  [unwired: 4 in, 3 out]
                  }
                }
                n425 = call "BORRADO_MEJORADO_Gonzalo.vi"("Bytes LIBRE OK"=w895, "Bytes Minimo de Memoria libre"=w896) -> ()  [unwired: 10 in]
                n426 = call "Borrar_carpeta.vi"("Nº Archivos Max"=w897, "Path Carpeta"=w901) -> ()  [unwired: 1 in]
                n427 = call "Comprimir_a_1_archivo.vi"("Acel_paths"=w900) -> ("path_Pasada"=→"created path":path)
              }
            }
            n428 = call <vilib>:"Watchdog Clear.vi"("error in (no error)"=w677, "watchdogID in"=w678) -> ("error out"=w676:errorcluster)  [unwired: 5 in]
            n429 = local read "RFID_Error"() -> (w688:errorcluster)
            n430 = Merge Errors(w697, w676) -> (w689:errorcluster)
            n431 = Merge Errors(w686, w688, w689) -> (w698:errorcluster)
            n432 = Unbundle By Name(w698) -> ("status"=w692:bool)
            n433 = Select(t="Descarga datos", s=FALSE, f="Espera") -> (s? t:f=w694:string)
            n434 = Select(t="TEST", s=w692, f=w694) -> (s? t:f=w691:string)
          }
          frame "TEST" {
            n435 = local read "Watchdog config"() -> (w916:T1)
            n436 = call <vilib>:"Watchdog Configure.vi"("expiration actions"=w916, "timeout (1 sec)"=200.0) -> ("error out"=w917:errorcluster, "watchdogID"=w914:u64)  [unwired: 4 in, 2 out]
            n437 = flat-sequence {
              tunnel: [w936] -> w921
              tunnel: w917 -> [w931]
              tunnel: w919 -> [w924]
              tunnel: [w949] -> w909
              tunnel: [w932] -> w918
              tunnel: w914 -> [w930]
              tunnel: [w929] -> w912
              tunnel: w913 -> [w926]
              tunnel: [w928] -> w911
              frame #0 {
                n438 = local read "Use Aura?"() -> (w922:bool)
                n439 = case shown="False" w922 {
                  tunnel: w926 -> [_ w957]
                  tunnel: [errorcluster {"status"=FALSE, "code"=0, "source"=""} ("error AURA") w952] -> w925
                  tunnel: w924 -> [_ w951]
                  frame False {
                  }
                  frame True {
                    n440 = local read "Parametros AuraWheel Health"() -> (w955:string[])
                    n441 = local read "RFID_LR6_Error"() -> (w963:errorcluster)
                    n442 = local read "T fuera rango"() -> (w961:bool)
                    n443 = local read "Max RMS Ruedas"() -> (w960:dbl[][])
                    n444 = local read "Problema WS"() -> (w959:bool)
                    n445 = local read "Fallo det presencia"() -> (w956:bool)
                    n446 = local read "RFID_Error"() -> (w962:errorcluster)
                    n447 = local read "LIMITE MAX"() -> (w954:dbl)
                    n448 = local read "LIMITE MIN"() -> (w953:dbl)
                    n449 = Not(x=w959) -> (.not. x?=w958:bool)
                    n450 = call "send_health_AURA.vi"("TEMPERATURA"=w961, "Parametros AuraWheel"=w955, "all rows"=w960, "WHEEL_SENSOR"=w958, "LIMITE MAX"=w954, "LIMITE MIN"=w953, "RFID_Error"=w962, "FOTOCELULA"=w956, "RFID_LR6_Error"=w963, "ESCRITURA ERROR"=w957, "FPGA ERROR"=w951) -> ("error AURA"=w952:errorcluster)  [unwired: 6 in, 2 out]
                  }
                }
                n451 = call <vilib>:"Watchdog Whack.vi"("error in (no error)"=w931, "reset watchdog after expire? (F)"=TRUE, "watchdogID in"=w930) -> ("error out"=w928:errorcluster, "watchdogID out"=w929:u64)  [unwired: 2 in, 1 out]
                n452 = Merge Errors(w924, w925) -> (w923:errorcluster)
                n453 = Get Date/Time In Seconds() -> (seconds since 1Jan1904=w943:timestamp)
                n454 = local read "Ultimo TEST"() -> (w944:timestamp)
                n455 = To Double Precision Float(number=w943) -> (double precision float=w945:dbl)
                n456 = Subtract(x=w945, y=3600.0) -> (x-y=w947:dbl)
                n457 = To Time Stamp(1:w947) -> (0:w948:timestamp)
                n458 = In Range and Coerce(upper limit=w943, x=w944, lower limit=w948) -> (In Range?=w942:bool)  [unwired: 1 out]
                n459 = case shown="False" w942 {
                  tunnel: w926 -> [w992 _]
                  tunnel: w923 -> [w968 w1007]
                  tunnel: [w977 errorcluster {"status"=FALSE, "code"=0, "source"=""} ("error out")] -> w949
                  tunnel: [w968 w1007] -> w932
                  frame False {
                    n460 = local read "Timeout ruedas"() -> (w969:bool)
                    n461 = local read "Aviso no detección"() -> (w975:string)
                    n462 = local read "Aviso temperatura"() -> (w974:string)
                    n463 = case shown="True" w969 {
                      selector: w969 -> [_ w1004]
                      tunnel: ["\r" w1005] -> w967
                      frame False {
                      }
                      frame True {
                        w994 = "\n"
                        n464 = local read "Nº Ruedas 1"() -> (w1001:i32)
                        n465 = local read "NºRuedas 2"() -> (w996:i32)
                        n466 = call "ErrorRuedas.vi"("Buffer Overflow"=w1004) -> ("error out"=w1006:errorcluster)
                        n467 = Number To Decimal String(number=w1001) -> (decimal integer string=w999:string)  [unwired: 1 in]
                        n468 = Number To Decimal String(number=w996) -> (decimal integer string=w995:string)  [unwired: 1 in]
                        n469 = Concatenate Strings("Error Wheel sensors", "\n", "WS1 (ruedas):", w999, w994, "WS2 (ruedas):", w995, w994) -> (w997:string)
                        n470 = call "Error.vi"("Error con..."=w997, "error comunicacion 2"=w1006) -> ("String"=w1005:string)
                      }
                    }
                    n471 = local read "RFID_Error"() -> (w971:errorcluster)
                    n472 = local read "RFID_LR6_Error"() -> (w965:errorcluster)
                    n473 = local read "DC OK"() -> (w973:string)
                    n474 = call "Cabecera.vi"() -> ("String"=w990:string)
                    n475 = call "Adquisicion.vi"("Aviso no detección"=w975) -> ("String"=w989:string)
                    n476 = call "Temperatura.vi"("Aviso temperatura"=w974) -> ("String"=w988:string)
                    n477 = call "Fuente.vi"("DC OK"=w973) -> ("String"=w987:string)
                    n478 = call "FPGA.vi"("error out"=w968) -> ("String"=w986:string)
                    n479 = call "Escritura.vi"("error out"=w992) -> ("String"=w985:string)
                    n480 = call "Error.vi"("Error con..."="Error con el lecto RFID NEM", "error comunicacion 2"=w971) -> ("String"=w970:string)
                    n481 = call "Error.vi"("Error con..."="Error con el lecto RFID LR6-HD", "error comunicacion 2"=w965) -> ("String"=w964:string)
                    n482 = Concatenate Strings(w990, w989, w988, w987, w986, w985, w970, w964, w967) -> (w991:string)
                    n483 = call "STRINGhorafechA(SubVI).vi"() -> ("STRINGhora_fecha"=w984:string)
                    n484 = Concatenate Strings(w984, ".txt" ("string")) -> (w980:string)
                    n485 = Get Date/Time In Seconds() -> (seconds since 1Jan1904=→"Ultimo TEST":timestamp)
                    n486 = Build Array("c", "TEST" ("element"), w980) -> (w982:string[])
                    n487 = Array of Strings to Path(0:w982) -> (2:w978:path)  [unwired: 1 out]
                    n488 = Write to Text File(file (use dialog)=w978, text=w991) -> (error out=w977:errorcluster)  [unwired: 1 in, 3 out]
                  }
                  frame True {
                  }
                }
                n489 = local read "Fallo det presencia"() -> (w935:bool)
                n490 = Unbundle By Name(w932) -> ("status"=w933:bool)
                n491 = local read "T fuera rango"() -> (w941:bool)
                n492 = Compound Arithmetic op=OR(w933, w935) -> (w934:bool)
                n493 = local write "Reset del controlador"(w934) -> ()
                n494 = Select(t="Escape", s=w941, f="Espera") -> (s? t:f=w938:string)
                n495 = Select(t="Configuracion", s=w934, f=w938) -> (s? t:f=w936:string)
              }
            }
            n496 = call <vilib>:"Watchdog Clear.vi"("error in (no error)"=w911, "watchdogID in"=w912) -> ("error out"=w910:errorcluster)  [unwired: 5 in]
            n497 = Merge Errors(w910, w909) -> (w908:errorcluster)
          }
        }
        "Estado" <- w84
        "error manipulacion archivos" <- w86
        n498 = local read "Parar la aplicación"() -> (w83:bool)
      }
      n499 = xnode "Close FPGA VI Reference"("FPGA VI Reference In"=w76, "error in"=w75) -> ("error out"=→"error FPGA":errorcluster)
    }
    frame #3 {
      n500 = local read "RFID_ID"() -> (w1011:refnum<k5>)
      n501 = call "LH6HD.vi"("Action"=enum16{"Init", "Start", "Read", "Stop", "Exit"}."Stop") -> ("error out"=→"RFID_LR6_Error":errorcluster)  [unwired: 9 in, 1 out]
      n502 = TCP Close Connection(connection ID=w1011) -> (error out=→"RFID_Error":errorcluster)  [unwired: 1 in, 2 out]
    }
  }
